vi "Experiment header-bundle parameters section wise.vi"(6 "Logging queue element":T1={"Imaging Protocol"=enum."Live Imaging", "Number of Trials"=0, "Frame Size"=100, "# Averaged frames"=0, "Dwell time (us)"=0.1, "Index of Z-plane"=0, "Timelapse?"=FALSE, "Logging process is active"=FALSE, "Speed logging enabled"=FALSE, "tdms file ref"=refnum, "path"=path "", "Trial Number"=0, "Expected # points acquired"=FALSE, "Manually stopped"=FALSE, "Last trial"=FALSE, "Ch0 data"=[], "Ch1 data"=[], "Ref Data"=[], "Ref Frame Time"=[], "Image Time"=[], "Continuous Time"=[], "Ref X Length"=0, "Ref Y Length"=0, "# Ref Averaged frames"=0, "Ref Dwell time (us)"=0.0, "Points acquired"={"Ch0 last trial"=0, "Ch1 last trial"=0, "All trials"=0}, "HW Timings File"=refnum} {"Ref Dwell time (us)" format="%#.6g"; "Frame Size" items=["100X100"=100, "128X128"=128, "200X200"=200, "256X256"=256, "512X512"=512, "1024x1024"=1024, "2048x2048"=2048]; "Dwell time (us)" format="%#.6g"}, 7 "Update header\ninterface cluster ?":bool, 8 "error in (no error)":errorcluster, 9 "Experiment data folder path":path, 10 "AOL_Globals":T25={"Imaging Protocol"=enum."AOL Z-Stack", "Number of POI"=0, "Number of Miniscans"=0, "Number of Trials"=0, "Number of Cycles "=0, "# Averaged Frames"=0, "Laser power (%)"=0, "Pockels (V)"=0.0, "Acquisition Length (sec)"=0.0, "Fill time (us)"=0.0, "POI Dwell time (us)"=0.0, "Miniscan Dwell time per pixel (us)"=0.0, "PMT 1"=0.0, "PMT 2"=0.0, "Back Apperture (mA)"=200.0, "Frame Size"=0, "Center Frequency"=0.0, "Field of View (um)"=175.0, "Field of View (norm)"=0.0, "DwellTime (us)"=0.0, "Ref Dwell Time (us)"=0.0, "Wavelength (nm)"=0.0, "Zoom"=0.0, "AOL Z"=0.0, "AOL Mode"=enum."Raster", "GridXY"=0.0, "GridZ"=0.0, "TriggerPeriod (sec)"=0.0, "Number of Pixels in Miniscan"=0, "Experiment folder path"=path "", "X centre"=0.0, "Y centre"=0.0, "Angle (degrees)"=0.0, "Angle Xs (degrees)"=0.0, "Angle Ys (degrees)"=0.0, "Plane Mode"=0, "Threshold"=[], "Regenerate Chirps"=FALSE, "Rectangle ROI length (pixels)"=0, "Rectangle ROI height (pixels)"=0, "AOD fill"=4900, "StartupDelay"=0, "Samples Wait after Trigger"=5080, "Slip Cycle"=600000, "Add Cycle"=TRUE, "Functional Mode"=enum."Point", "Z Start"=0.0, "Z Stop"=0.0, "# Planes"=0, "Total Pixels"=0, "Variable Miniscan Pixels"=[], "Use Variable Length"=FALSE, "Use Variable Resolution"=FALSE, "Laser power (%) at Z Start"=0, "Laser power (%) at Z Stop"=0, "Ref Z Step"=0} {"Angle Ys (degrees)" format="%#.6g"; "Angle Xs (degrees)" format="%#.6g"; "Plane Mode" items=["XY Plane", "XZ Plane", "YZ Plane", "arbitraryplane"]; "Frame Size" items=["100X100"=100, "128X128"=128, "200X200"=200, "256X256"=256, "512X512"=512, "1024x1024"=1024, "2048x2048"=2048]; "Back Apperture (mA)" format="%#.6g"; "Pockels (V)" format="%#.6g"; "PMT 2" format="%#.6g"; "PMT 1" format="%#.6g"; "Angle (degrees)" format="%#.6g"; "POI Dwell time (us)" format="%#.6g"}, 11 "Header file sections":T5=enum."GLOBAL PARAMETERS") -> (0 "error out":errorcluster, 3 "All header parameters in":T6 {"VOLUME IMAGING"."Plane Mode" items=["XY Plane", "XZ Plane", "YZ Plane", "arbitraryplane"]; "VOLUME IMAGING"."Basic Image meta data"."Frame Size" items=["100X100"=100, "128X128"=128, "200X200"=200, "256X256"=256, "512X512"=512, "1024x1024"=1024, "2048x2048"=2048]; "AOL Z-STACK"."Hdr Basic Image meta data"."Frame Size" items=["100X100"=100, "128X128"=128, "200X200"=200, "256X256"=256, "512X512"=512, "1024x1024"=1024, "2048x2048"=2048]; "MOTOR Z-STACK"."Hdr Basic Image meta data"."Frame Size" items=["100X100"=100, "128X128"=128, "200X200"=200, "256X256"=256, "512X512"=512, "1024x1024"=1024, "2048x2048"=2048]; "FUNCTIONAL IMAGING"."Plane Mode" items=["XY Plane", "XZ Plane", "YZ Plane", "arbitraryplane"]; "FUNCTIONAL IMAGING"."Basic Image meta data"."Frame Size" items=["100X100"=100, "128X128"=128, "200X200"=200, "256X256"=256, "512X512"=512, "1024x1024"=1024, "2048x2048"=2048]; "TIME SERIES"."Basic Image meta data"."Frame Size" items=["100X100"=100, "128X128"=128, "200X200"=200, "256X256"=256, "512X512"=512, "1024x1024"=1024, "2048x2048"=2048]})   [LabVIEW 2020]
uses:
  Typedefs/Controls/AOL_Globals.ctl
  Typedefs/Imaging Protocols enum.ctl
  Typedefs/Frame Size.ctl
  Typedefs/AOL modes.ctl
  Typedefs/Plane Mode.ctl
  Typedefs/Functional Mode.ctl
  Typedefs/Header parameters cluster-ALL.ctl
  Typedefs/Header subclusters/Header params -Login.ctl
  Typedefs/Header subclusters/Header params-Global Parameters.ctl
  Misc/Experiment Type.ctl
  Typedefs/Header subclusters/Header params-Imaging Modes.ctl
  Typedefs/Header subclusters/Header params-Time Series.ctl
  Typedefs/Header subclusters/Header params-Basic image meta data.ctl
  Typedefs/Header subclusters/Header params-Motor Z-stack.ctl
  Typedefs/Header subclusters/Header params-AOL Z-stack.ctl
  Typedefs/Header subclusters/Header params-Functional Imaging.ctl
  Typedefs/Header subclusters/Header params-Movement correction.ctl
  Typedefs/Reference source.ctl
  Typedefs/Header subclusters/Header params-Calibration Setup.ctl
  Typedefs/Header subclusters/Header params-statistics.ctl
  Misc/Biology Information.ctl
  Typedefs/Header subclusters/Header params-calibration data.ctl
  Typedefs/Header file sections.ctl
  Typedefs/Logging queue element.ctl
  Typedefs/Acquired points count.ctl
  ROI Entry screen/Typedefs/FGV ROI Time Ops.ctl
  Typedefs/Header file interface module functions enum.ctl
  Global Variables/General Globals.vi
  User profiles code/Globals/gl_UsrProfiles globals.vi
  Global Variables/gl_UI Ctrl Refs.vi
  Peripherals Control/Pockels/Globals/gl_Pockels control globals.vi
  Global Variables/gl_RefPlotRefreshRate.vi
  Configuration code/Calibration/Globals/gl_Calibration globals.vi
  Typedefs/Header subclusters/Header params-Volume Imaging.ctl
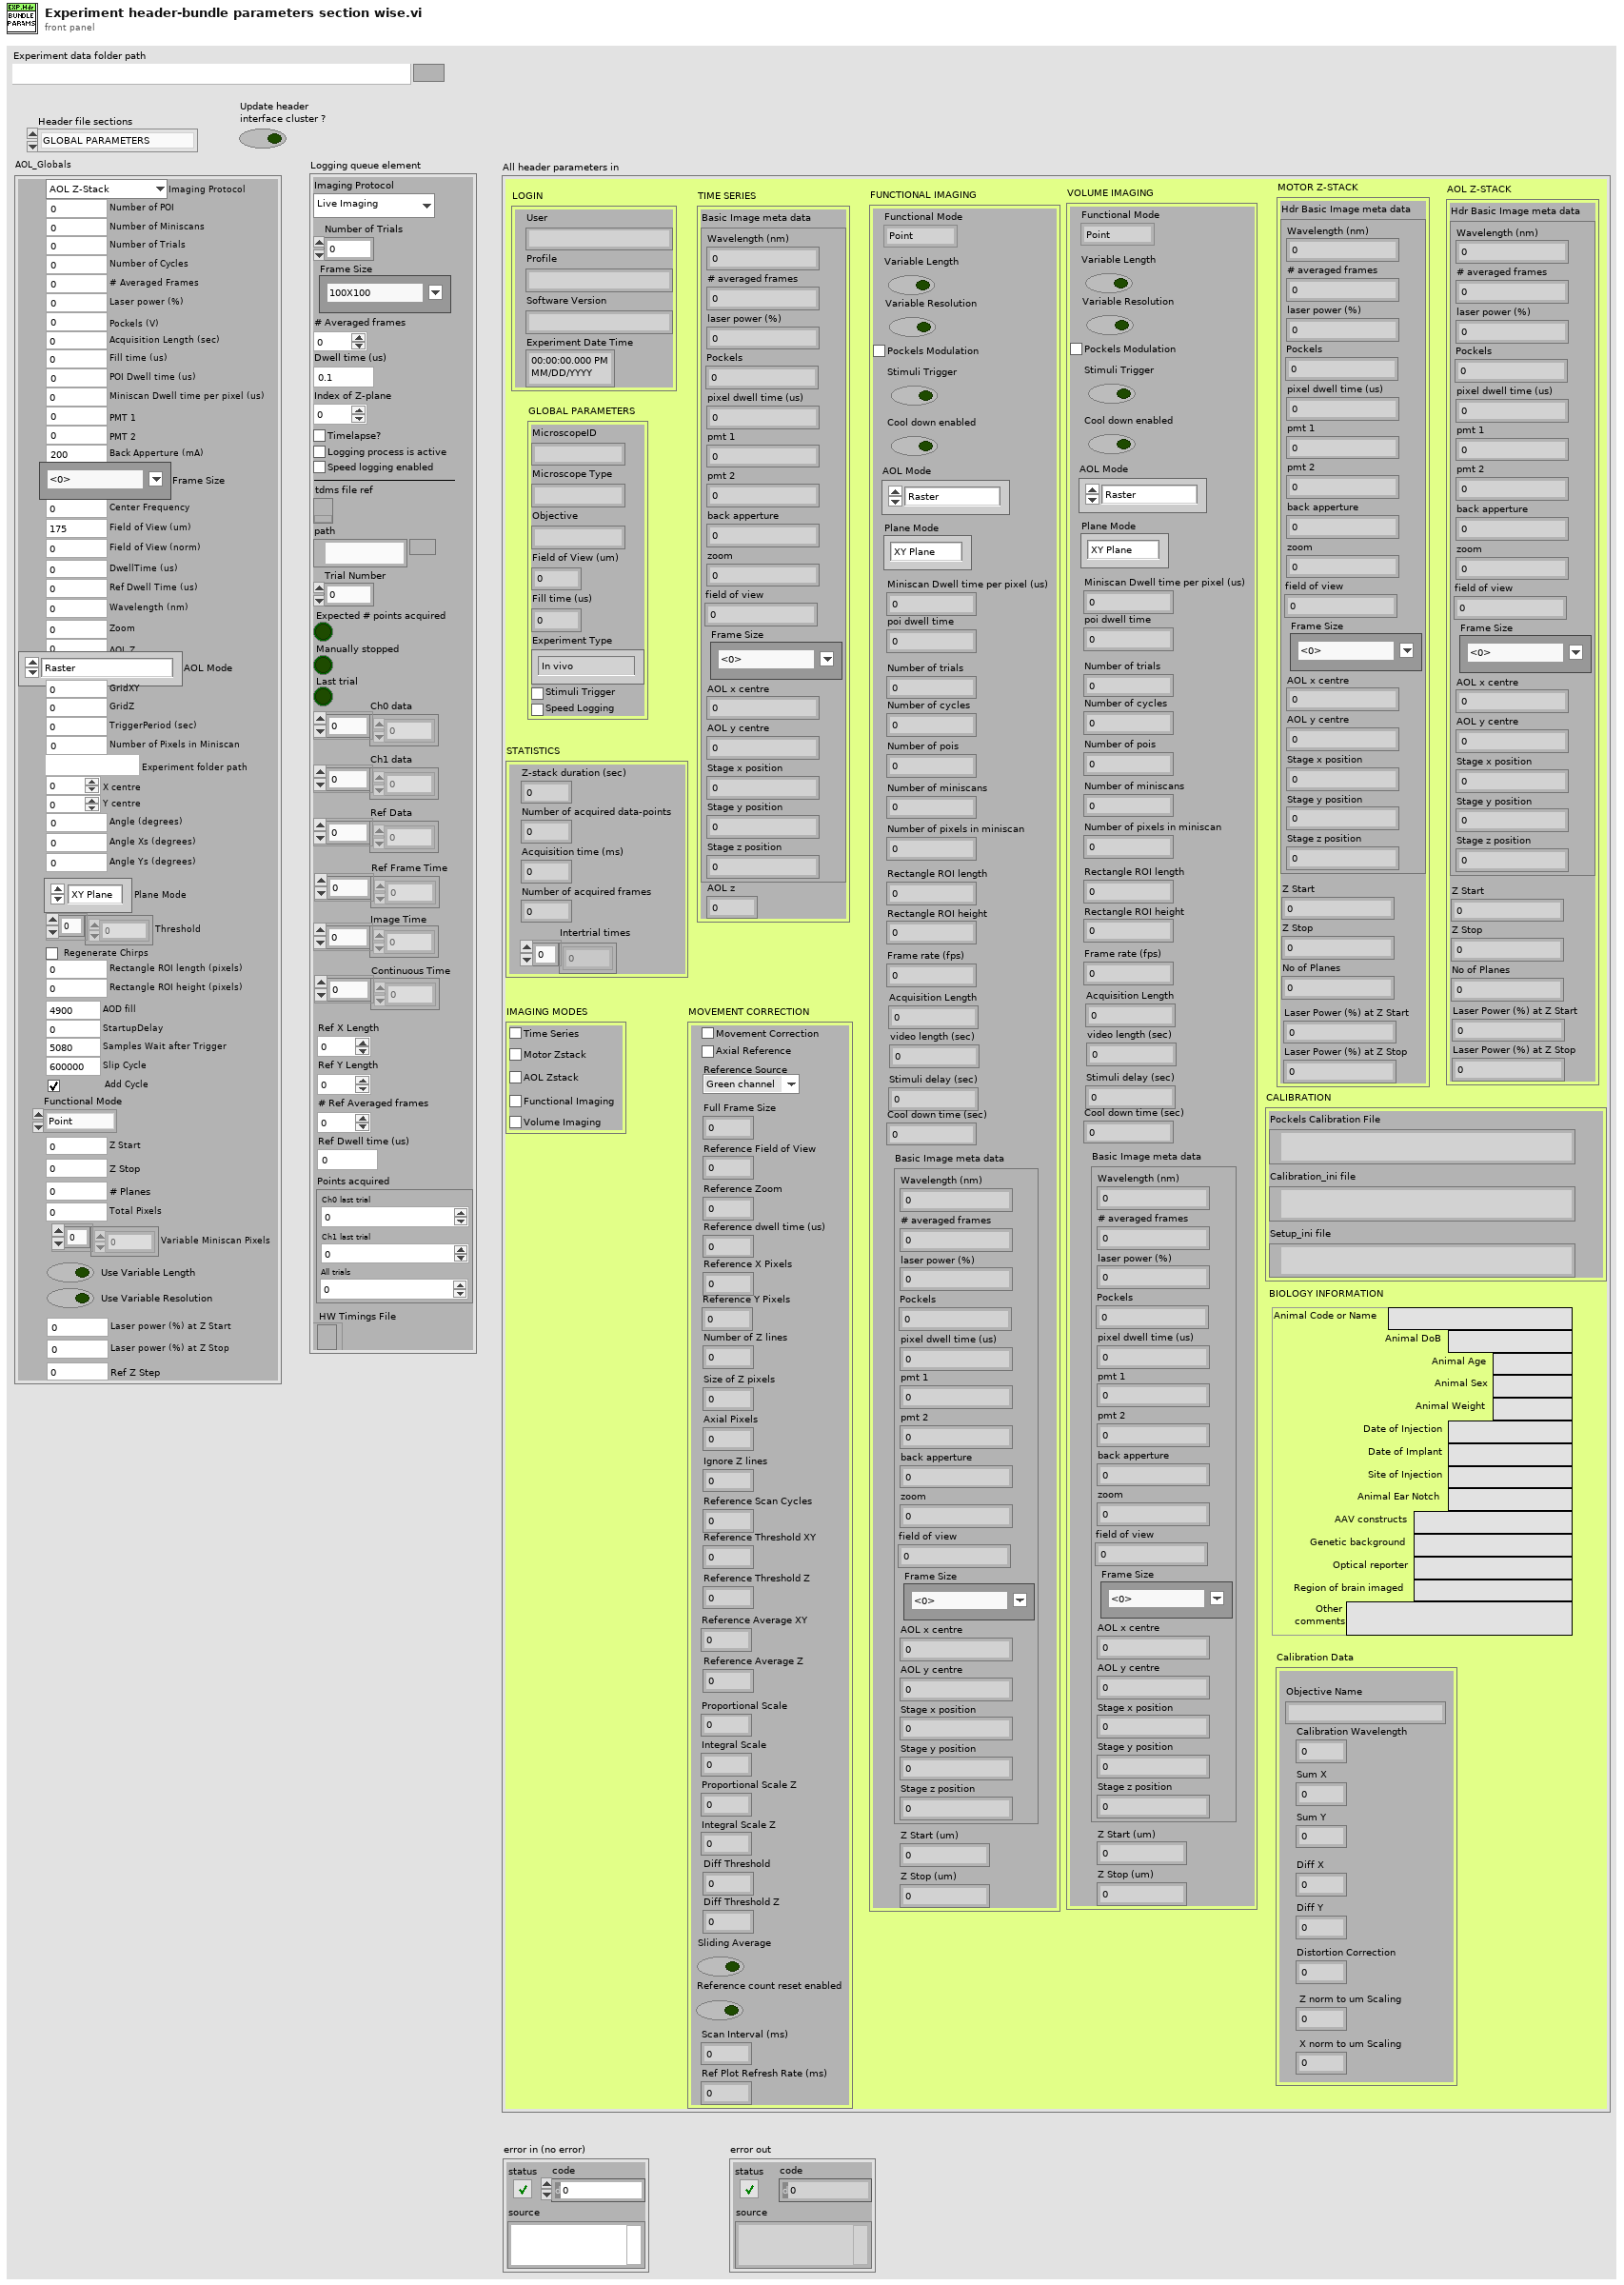
[diagram p1: front panel]
types:
  T1 = typedef "Logging queue element.ctl" = cluster{"Imaging Protocol":T2, "Number of Trials":u16, "Frame Size":T3, "# Averaged frames":u16, "Dwell time (us)":dbl, "Index of Z-plane":i32, "Timelapse?":bool, "Logging process is active":bool, "Speed logging enabled":bool, "tdms file ref":refnum<k34>, "path":path, "Trial Number":i32, "Expected # points acquired":bool, "Manually stopped":bool, "Last trial":bool, "Ch0 data":u32[], "Ch1 data":u32[], "Ref Data":u32[], "Ref Frame Time":u64[], "Image Time":u64[], "Continuous Time":u64[], "Ref X Length":u16, "Ref Y Length":u16, "# Ref Averaged frames":u16, "Ref Dwell time (us)":dbl, "Points acquired":T4, "HW Timings File":refnum<file>}
  T2 = typedef "Imaging Protocols enum.ctl" = enum16{"AOL Z-Stack", "Motor Z Stack", "Parameter Sweep", "Functional Acquisition", "Single Plane Acquisition", "Volume Acquisition", "Live Imaging", "Live Plane Imaging", "Live Volume Imaging"}
  T3 = typedef "Frame Size.ctl" = u16
  T4 = typedef "Acquired points count.ctl" = cluster{"Ch0 last trial":u64, "Ch1 last trial":u64, "All trials":u64}
  T5 = typedef "Header file sections.ctl" = enum16{"ALL SECTIONS", "LOGIN", "GLOBAL PARAMETERS", "CALIBRATION DATA", "IMAGING MODES", "TIME SERIES", "MOTOR Z-STACK", "AOL Z-STACK", "FUNCTIONAL IMAGING", "VOLUME IMAGING", "MOVEMENT CORRECTION", "CALIBRATION", "STATISTICS", "BIOLOGY INFORMATION"}
  T6 = typedef "Header parameters cluster-ALL.ctl" = cluster{"LOGIN":T7, "GLOBAL PARAMETERS":T8, "IMAGING MODES":T10, "TIME SERIES":T11, "MOTOR Z-STACK ":T13, "AOL Z-STACK":T14, "FUNCTIONAL IMAGING":T15, "VOLUME IMAGING":T15, "MOVEMENT CORRECTION":T19, "CALIBRATION":T21, "STATISTICS":T22, "BIOLOGY INFORMATION":T23, "Calibration Data":T24}
  T7 = typedef "Header params -Login.ctl" = cluster{"User":string, "Profile":string, "Software Version":string, "Experiment Date Time":timestamp}
  T8 = typedef "Header params-Global Parameters.ctl" = cluster{"MicroscopeID":string, "Microscope Type":string, "Objective":string, "Field of View (um)":dbl, "Fill time (us)":dbl, "Experiment Type":T9, "Stimuli Trigger":bool, "Speed Logging":bool}
  T9 = typedef "Experiment Type.ctl" = enum16{"In vivo", "In vitro", "Testing", "Calibration", "Other"}
  T10 = typedef "Header params-Imaging Modes.ctl" = cluster{"Time Series":bool, "Motor Zstack":bool, "AOL Zstack":bool, "Functional Imaging":bool, "Volume Imaging":bool}
  T11 = typedef "Header params-Time Series.ctl" = cluster{"Basic Image meta data":T12, "AOL z":dbl}
  T12 = typedef "Header params-Basic image meta data.ctl" = cluster{"Wavelength (nm)":dbl, "# averaged frames":dbl, "laser power (%)":dbl, "Pockels":dbl, "pixel dwell time (us)":dbl, "pmt 1":dbl, "pmt 2":dbl, "back apperture":dbl, "zoom":dbl, "field of view":dbl, "Frame Size":T3, "AOL x centre":dbl, "AOL y centre":dbl, "Stage x position":dbl, "Stage y position":dbl, "Stage z position":dbl}
  T13 = typedef "Header params-Motor Z-stack.ctl" = cluster{"Hdr Basic Image meta data":T12, "Z Start":dbl, "Z Stop":dbl, "No of Planes":i32, "Laser Power (%) at Z Start":dbl, "Laser Power (%) at Z Stop":dbl}
  T14 = typedef "Header params-AOL Z-stack.ctl" = cluster{"Hdr Basic Image meta data":T12, "Z Start":dbl, "Z Stop":dbl, "No of Planes":i32, "Laser Power (%) at Z Start":dbl, "Laser Power (%) at Z Stop":dbl}
  T15 = typedef "Header params-Functional Imaging.ctl" = cluster{"Functional Mode":T16, "Variable Length":bool, "Variable Resolution":bool, "Pockels Modulation":bool, "Stimuli Trigger":bool, "Cool down enabled":bool, "AOL Mode":T17, "Plane Mode":T18, "Miniscan Dwell time per pixel (us)":dbl, "poi dwell time":dbl, "Number of trials":dbl, "Number of cycles":dbl, "Number of pois":dbl, "Number of miniscans":dbl, "Number of pixels in miniscan":dbl, "Rectangle ROI length":dbl, "Rectangle ROI height":dbl, "Frame rate (fps)":dbl, "Acquisition Length":dbl, "video length (sec)":dbl, "Stimuli delay (sec)":dbl, "Cool down time (sec)":dbl, "Basic Image meta data":T12, "Z Start (um)":dbl, "Z Stop (um)":dbl}
  T16 = typedef "Functional Mode.ctl" = enum16{"Point", "Line", "Patch", "Plane", "Volume"}
  T17 = typedef "AOL modes.ctl" = enum16{"Raster", "Structural", "Pointing", "Mini Scan", "Alignment"}
  T18 = typedef "Plane Mode.ctl" = u16
  T19 = typedef "Header params-Movement correction.ctl" = cluster{"Movement Correction":bool, "Axial Reference":bool, "Reference Source":T20, "Full Frame Size":dbl, "Reference Field of View":dbl, "Reference Zoom":dbl, "Reference dwell time (us)":dbl, "Reference X Pixels":dbl, "Reference Y Pixels":dbl, "Number of Z lines":dbl, "Size of Z pixels":dbl, "Axial Pixels":dbl, "Ignore Z lines":dbl, "Reference Scan Cycles":dbl, "Reference Threshold XY":dbl, "Reference Threshold Z":dbl, "Reference Average XY":dbl, "Reference Average Z":dbl, "Proportional Scale":dbl, "Integral Scale":dbl, "Proportional Scale Z":dbl, "Integral Scale Z":dbl, "Diff Threshold":dbl, "Diff Threshold Z":dbl, "Sliding Average":bool, "Reference count reset enabled":bool, "Scan Interval (ms)":dbl, "Ref Plot Refresh Rate (ms)":dbl}
  T20 = typedef "Reference source.ctl" = enum16{"Green channel", "Red channel"}
  T21 = typedef "Header params-Calibration Setup.ctl" = cluster{"Pockels Calibration File":path, "Calibration_ini file":path, "Setup_ini file":path}
  T22 = typedef "Header params-statistics.ctl" = cluster{"Z-stack duration (sec)":dbl, "Number of acquired data-points":dbl, "Acquisition time (ms)":dbl, "Number of acquired frames":dbl, "Intertrial times":dbl[]}
  T23 = typedef "Biology Information.ctl" = cluster{"Animal Code or Name":string, "Animal DoB":string, "Animal Age":string, "Animal Sex":string, "Animal Weight":string, "Date of Injection":string, "Date of Implant":string, "Site of Injection":string, "Animal Ear Notch":string, "AAV constructs":string, "Genetic background":string, "Optical reporter":string, "Region of brain imaged":string, "Other \ncomments":string}
  T24 = typedef "Header params-calibration data.ctl" = cluster{"Objective Name":string, "Calibration Wavelength":dbl, "Sum X":dbl, "Sum Y":dbl, "Diff X":dbl, "Diff Y":dbl, "Distortion Correction":dbl, " Z norm to um Scaling":dbl, " X norm to um Scaling":dbl}
  T25 = typedef "AOL_Globals.ctl" = cluster{"Imaging Protocol":T2, "Number of POI":u16, "Number of Miniscans":u16, "Number of Trials":u16, "Number of Cycles ":u64, "# Averaged Frames":u16, "Laser power (%)":u8, "Pockels (V)":dbl, "Acquisition Length (sec)":dbl, "Fill time (us)":dbl, "POI Dwell time (us)":dbl, "Miniscan Dwell time per pixel (us)":dbl, "PMT 1":dbl, "PMT 2":dbl, "Back Apperture (mA)":dbl, "Frame Size":T3, "Center Frequency":dbl, "Field of View (um)":dbl, "Field of View (norm)":dbl, "DwellTime (us)":dbl, "Ref Dwell Time (us)":dbl, "Wavelength (nm)":dbl, "Zoom":dbl, "AOL Z":dbl, "AOL Mode":T17, "GridXY":dbl, "GridZ":dbl, "TriggerPeriod (sec)":dbl, "Number of Pixels in Miniscan":u16, "Experiment folder path":path, "X centre":dbl, "Y centre":dbl, "Angle (degrees)":dbl, "Angle Xs (degrees)":dbl, "Angle Ys (degrees)":dbl, "Plane Mode":T18, "Threshold":u16[], "Regenerate Chirps":bool, "Rectangle ROI length (pixels)":u16, "Rectangle ROI height (pixels)":u16, "AOD fill":u16, "StartupDelay":i32, "Samples Wait after Trigger":u16, "Slip Cycle":u32, "Add Cycle":bool, "Functional Mode":T16, "Z Start":dbl, "Z Stop":dbl, "# Planes":i32, "Total Pixels":i32, "Variable Miniscan Pixels":u16[], "Use Variable Length":bool, "Use Variable Resolution":bool, "Laser power (%) at Z Start":u8, "Laser power (%) at Z Stop":u8, "Ref Z Step":i8}
  T26 = typedef "FGV ROI Time Ops.ctl" = enum16{"Read", "Write Cycle Time", "Write Cycle Rate"}
  T27 = typedef "UI ctrl refs cluster.ctl" = cluster{"Top level VI path":path, "Top level VI ref":refnum<vi>, "User menu ref":refnum<k9>, "Sub Panel control":refnum<vi>, "Imaging Param Tab":refnum<vi>, "Occurrence-Start drivers":refnum<k4>, "Occurrence-Speed logging initialised":refnum<k4>, "Occurrence-XYZ stage initialised":refnum<k4>, "Exit button":refnum<vi>, "Status ind":refnum<vi>, "Set as origin":refnum<vi>, "Speed Logging":refnum<vi>, "Time Lapse":refnum<vi>, "Live Imaging":refnum<vi>, "AOL Z Stack":refnum<vi>, "Motor Z Stack":refnum<vi>, "Funct Acq button":refnum<vi>, "Hard Shutter":refnum<vi>, "Virtual Shutter":refnum<vi>, "Laser Power":refnum<vi>, "AOL Mode":refnum<vi>, "Frame Size":refnum<vi>, "Field of View":refnum<vi>, "Dwell Time":refnum<vi>, "Zoom":refnum<vi>, "AOL Z":refnum<vi>, "Objective":refnum<vi>, "Axis":refnum<vi>, "Paths & Names":refnum<vi>, "Experiment folder path (ind.)":refnum<vi>, "Last State (Ind.)":refnum<vi>, "Averages":refnum<vi>, "Angle (degrees)":refnum<vi>, "X centre":refnum<vi>, "Y centre":refnum<vi>, "Plane Mode":refnum<vi>, "# Planes":refnum<vi>, "Z Start":refnum<vi>, "Z Stop":refnum<vi>, "Z Step":refnum<vi>, "PMT 1":refnum<vi>, "PMT 2":refnum<vi>, "Stage XYZ Position":refnum<vi>, "Pockels@Z Start":refnum<vi>, "Pockels@Z Stop":refnum<vi>, "Obtain Z Start":refnum<vi>, "Obtain Z Stop":refnum<vi>, "Live stim.trig.period":refnum<vi>, "Live stim.trig.enable":refnum<vi>, "Movement Correction":refnum<vi>, "Load Reference Image":refnum<vi>, "XY Stage Move":refnum<vi>, "MovCor Cluster":refnum<vi>, "RefDAQParam":refnum<vi>, "Funct. Acq. Pockels Modulation":refnum<vi>, "Ref Laser Power":refnum<vi>, "Enable Video Recording":refnum<vi>, "Video Record-Live Imaging":refnum<vi>, "Video Record-Funct acq":refnum<vi>, "Reference Source":refnum<vi>, "AOL Z-stack Chirps Ready (ind)":refnum<vi>, "Target time between mov.cor. ref triggers (ms)":refnum<vi>, "Funct. Acq. Ref frame save":refnum<vi>, "Tracking button":refnum<vi>, "Show ref plots window":refnum<vi>, "Center freq ind (nm)":refnum<vi>, "Pickup mode (ind)":refnum<vi>, "Logging queue (ind)":refnum<vi>, "Back aperture power (ind.)":refnum<vi>, "Power after objective (ind.)":refnum<vi>, "Switch user":refnum<vi>, "Ls1 Conn. Status":refnum<vi>, "Ls1Tuning Status":refnum<vi>, "Ls1 Faults":refnum<vi>, "Ls1 Connection":refnum<vi>, "Ls1 Mode":refnum<vi>, "Ls1 POWER [mW]":refnum<vi>, "Ls1Shutter":refnum<vi>, "Ls1 Wavelength":refnum<vi>, "Ls1 Note":refnum<vi>, "Ls1 Confirm Wav":refnum<vi>, "Ls1 PreChrp Prism1":refnum<vi>, "Ls1 PreChrp Prism2":refnum<vi>, "Ls1 wav top Ind":refnum<vi>, "Ls1 power top Ind":refnum<vi>, "Ls1 Pump peak Hold":refnum<vi>, "Ls1 Status Ind":refnum<vi>, "Ls1 wav cancel":refnum<vi>, "Experiment Type":refnum<vi>, "Biology Information":refnum<vi>, "Camera recording status":refnum<vi>, "Optimise Obj. Pos.":refnum<vi>}
  T28 = typedef "Objective Config.ctl" = cluster{"Name":string, "Sum X":dbl, "Sum Y":dbl, "Diff X":dbl, "Diff Y":dbl, "Distortion Correction":dbl, "Z_norm to um_scaling":dbl, "X_norm to um_scaling":dbl, "Calibrated Wavelength":dbl}
  T29 = typedef "Header params-Volume Imaging.ctl" = cluster{"Functional Mode":T16, "Pockels Modulation":bool, "Number of pois":dbl, "Number of miniscans":dbl, "Number of cycles":dbl, "Number of trials":dbl, "Miniscan dwell time per pixel (us)":dbl, "Number of pixels in miniscan":dbl, "poi dwell time":dbl, "Rectangle ROI length":dbl, "Rectangle ROI height":dbl, "AOL Mode":T17, "Plane Mode":T18, "video length (sec)":dbl, "Frame rate (fps)":dbl, "Stimuli Timing (usec)":dbl, "Acquisition Length":dbl, "Basic Image meta data":T12, "Z Start (um)":dbl, "Z Stop (um)":dbl}
  T30 = typedef "Ref DAQ Param.ctl" = cluster{"Full Frame Size":u16, "Ref Field of View":sgl, "Ref Zoom":i8, "Ref_dwellTime":sgl, "Ref X-pixels-per-line(Npxr)":i16, "Ref Y-lines-per-image(Npyr)":i16, "Ref Z-lines-per-image":i16, "Ignore Z lines":i16, "Ref Scan Cycles":i32, "Ref threshold XY":u16, "Ref threshold Z":u16, "Ref average XY":u16, "Ref Average  Z":u16, "Proportional_scale":fxp<+,16,2>, "Integral_scale":fxp<+/-,16,12>, "Proportional_scale Z":fxp<+,16,2>, "Integral_scale Z":fxp<+/-,16,12>, "Diff_threshold":fxp<+,16,2>, "Diff_threshold _z":fxp<+,16,2>, "Sliding Average":bool, "Ref count reset enabled":bool, "Auto-centering":bool}
  T31 = typedef "Reference_Globals.ctl" = cluster{"Refrence data path":path, "Reference Rectangle":i16[][], "AOL Z":dbl, "No of pixels in a miniscan ":i32[], "Threshold":i16[], "No of miniscans":i32[], "Full Frame Size":u16, "Reference Image":T32, "dwelltime":dbl, "Zoom":dbl, "Field of View":dbl, "Z Step":i8, "Z pixels":i32, "Z Lines":u8, "Z Ignore":u8, "Laser":u8, "Auto centering":bool}
  T32 = typedef "IMAQ Image.ctl" = refnum<image>
  T33 = typedef "Header file interface module functions enum.ctl" = enum16{"Load experiment header file", "Save experiment header file", "Clear stored values", "Read stored values", "Update specific value in memory", "Update values in memory"}
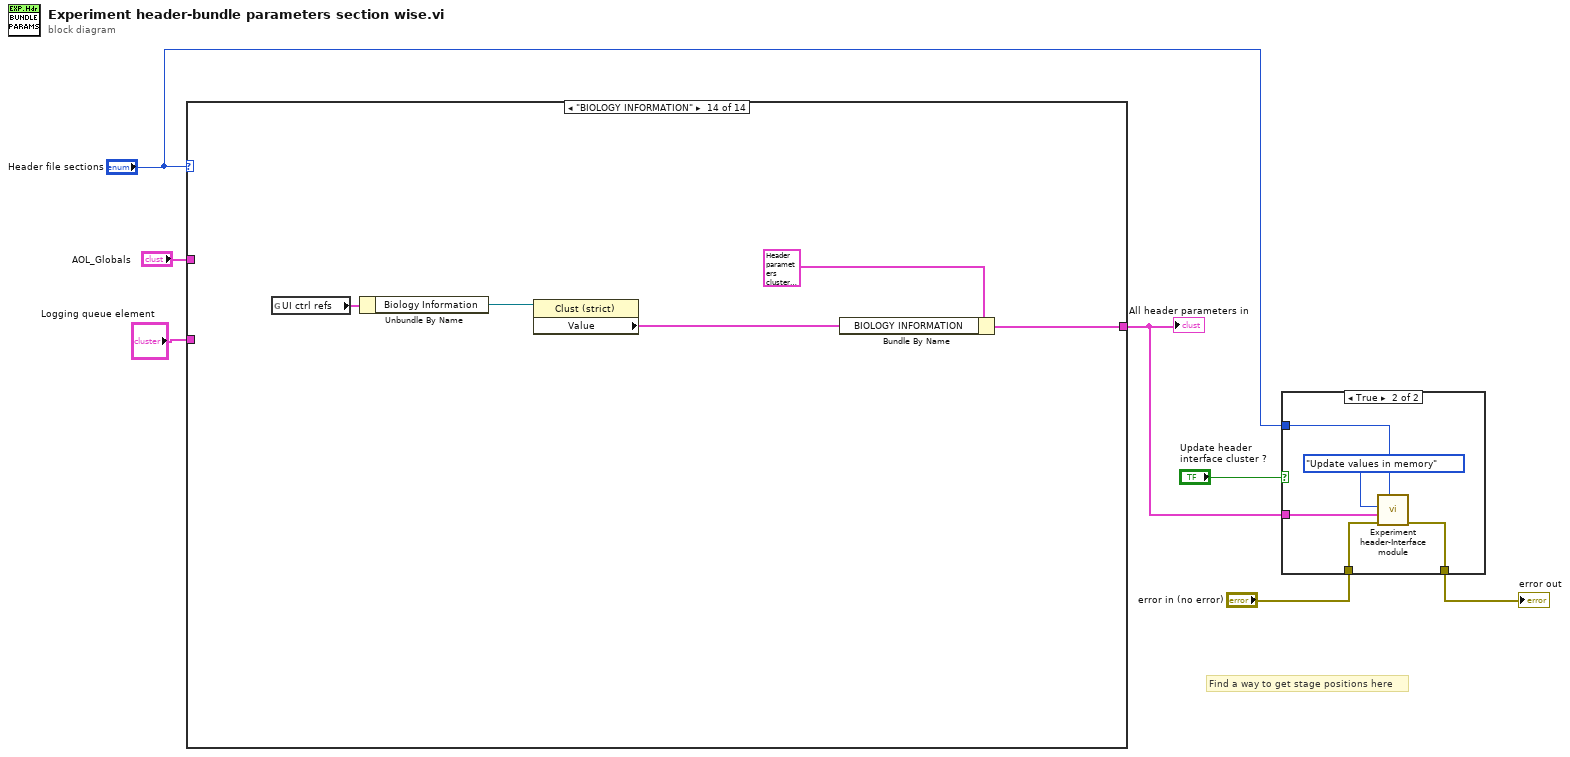
[diagram p0: block diagram]
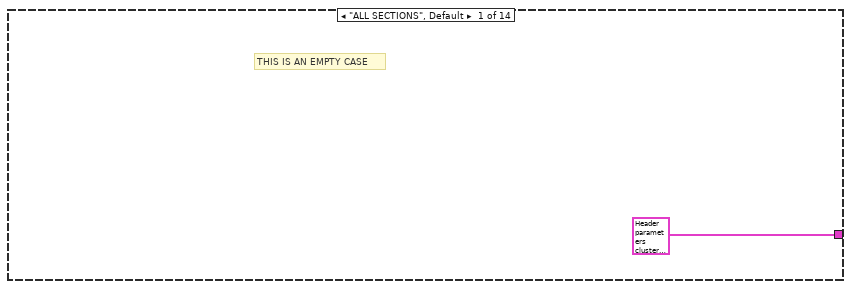
[diagram p3: hidden frame]
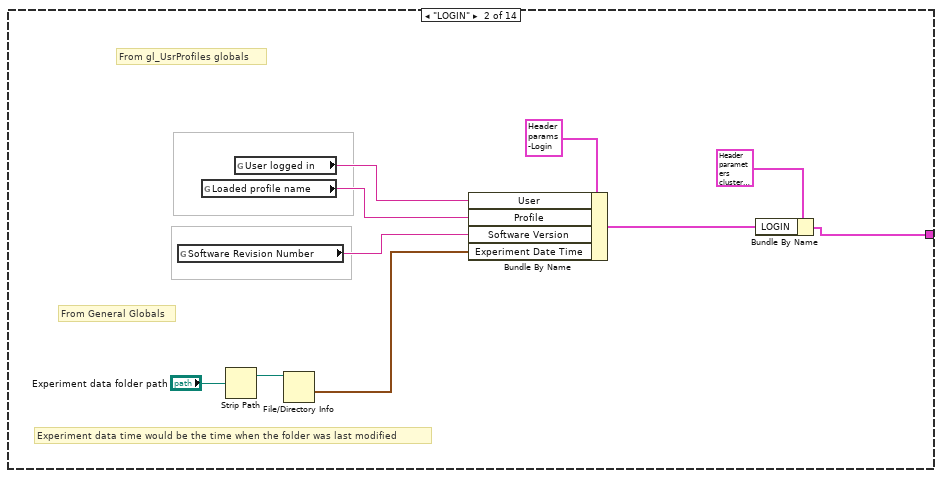
[diagram p4: hidden frame]
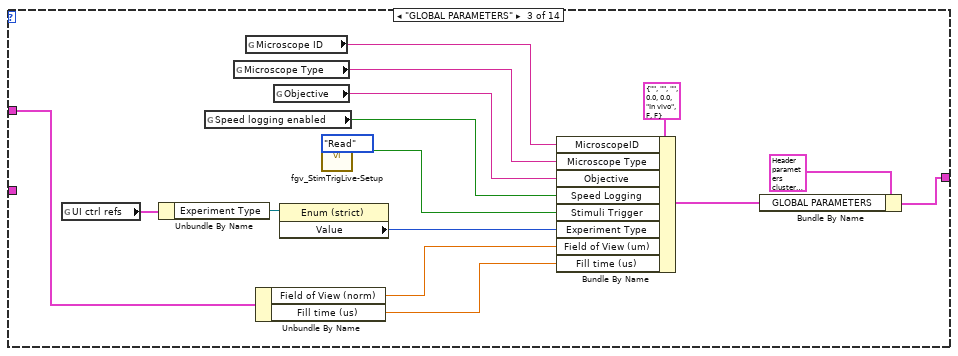
[diagram p5: hidden frame]
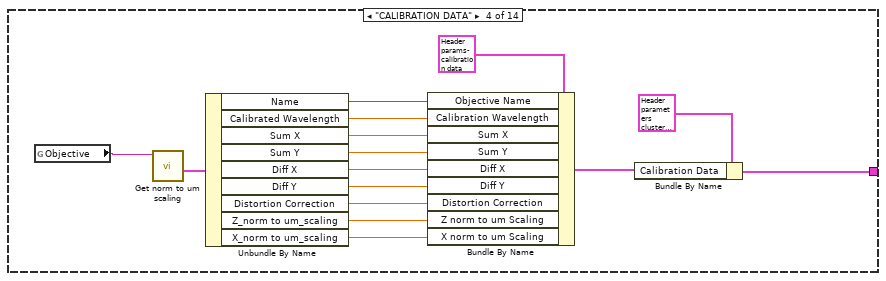
[diagram p6: hidden frame]
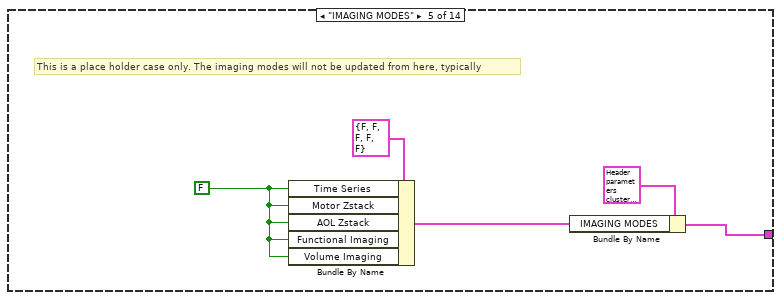
[diagram p7: hidden frame]
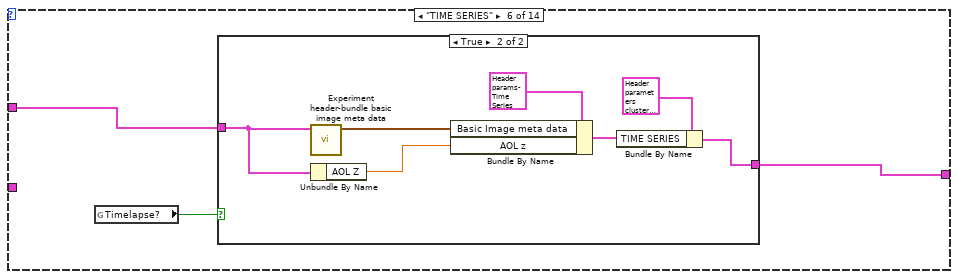
[diagram p8: hidden frame]
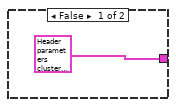
[diagram p9: hidden frame]
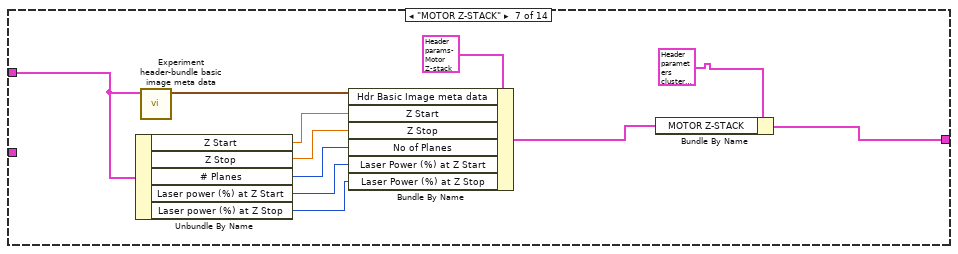
[diagram p10: hidden frame]
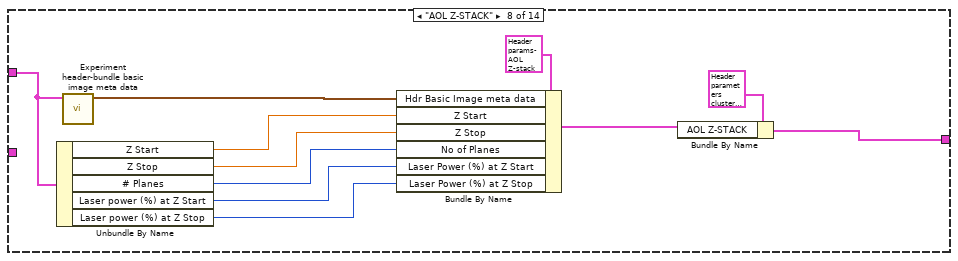
[diagram p11: hidden frame]
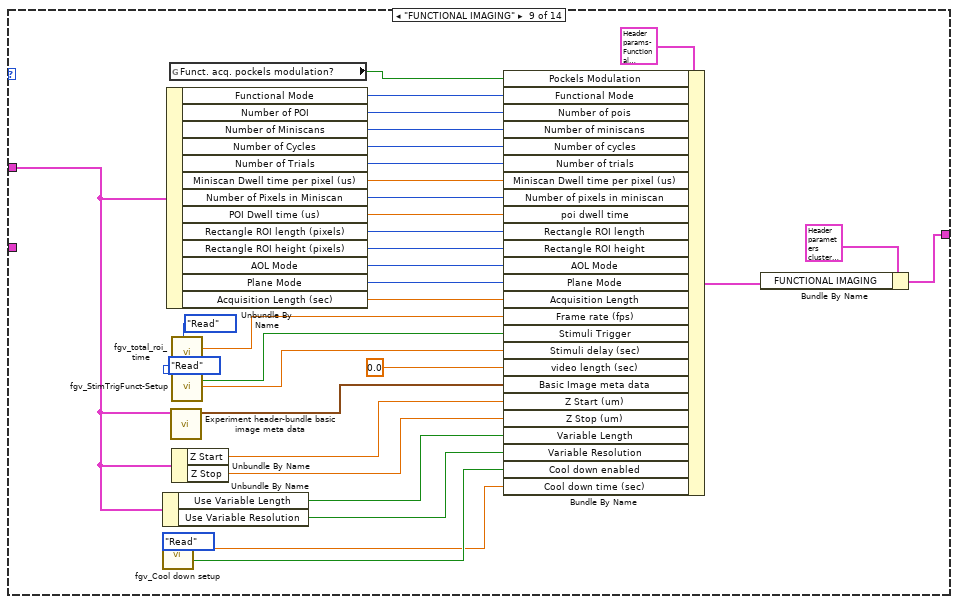
[diagram p12: hidden frame]
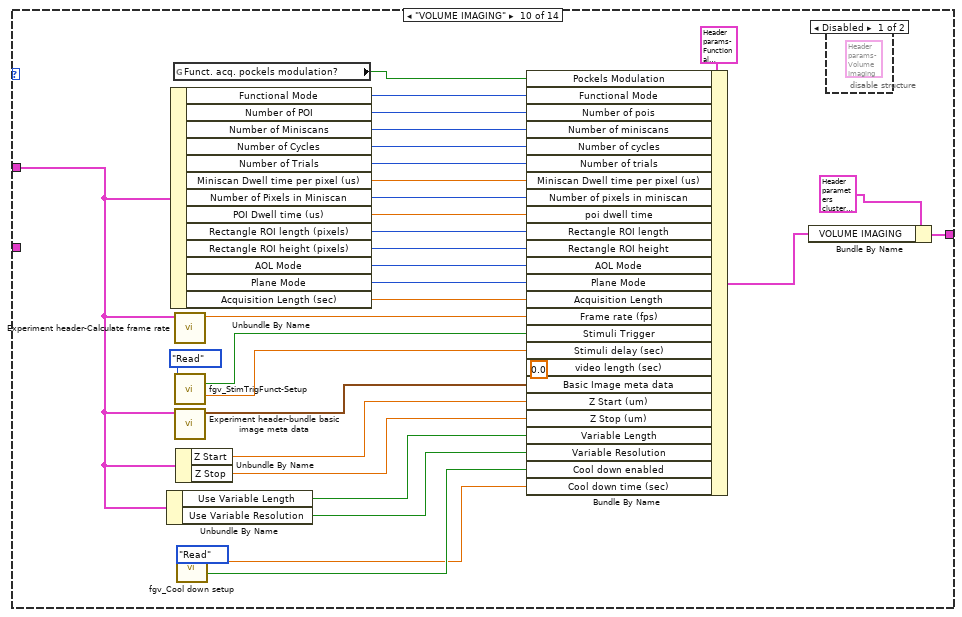
[diagram p13: hidden frame]
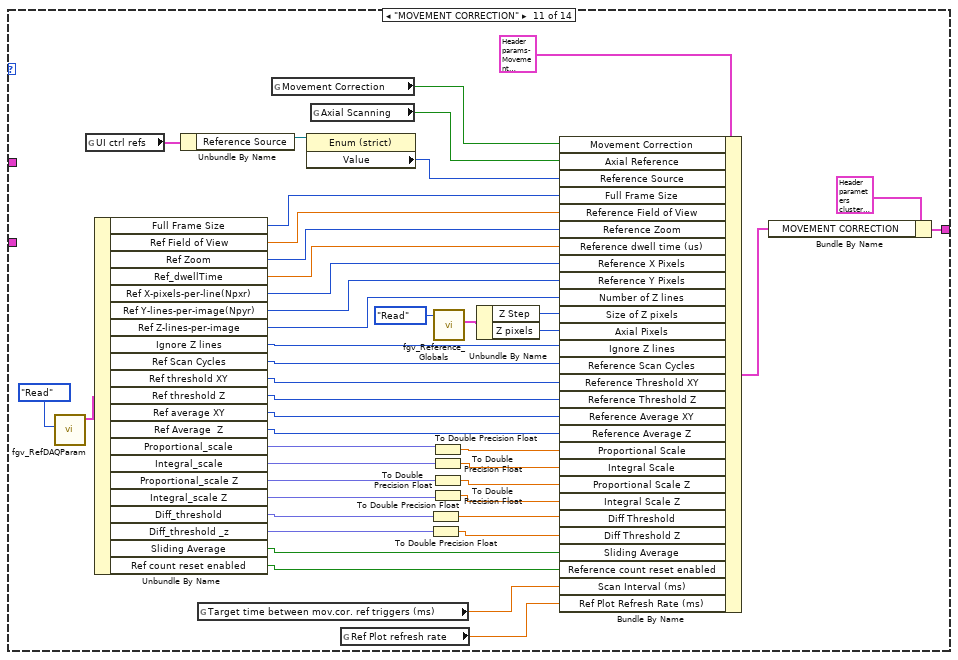
[diagram p15: hidden frame]
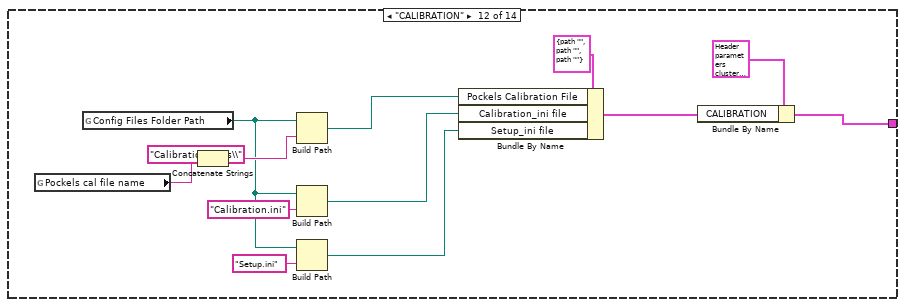
[diagram p16: hidden frame]
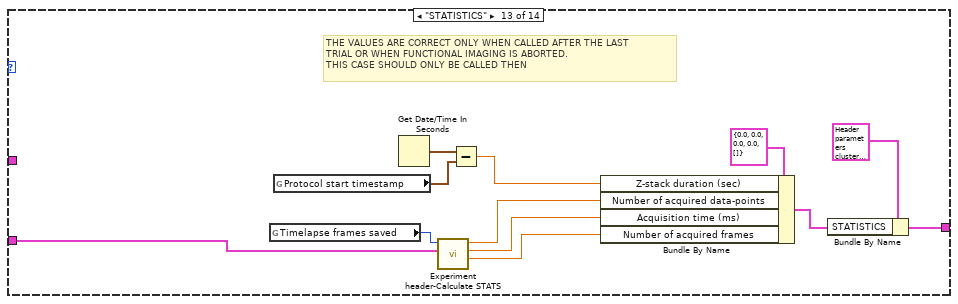
[diagram p17: hidden frame]
diagram:
  # "Find a way to get stage positions here"
  n1 = case shown="\"BIOLOGY INFORMATION\"" "Header file sections" {
    tunnel: "AOL_Globals" -> [_ _ w30 _ _ w56 w72 w83 w99 w130 _ _ _ _]
    tunnel: [T6 {"LOGIN"={"User"="", "Profile"="", "Software Version"="", "Experiment Date Time"=timestamp(0 s since 1904-01-01)}, "GLOBAL PARAMETERS"={"MicroscopeID"="", "Microscope Type"="", "Objective"="", "Field of View (um)"=0.0, "Fill time (us)"=0.0, "Experiment Type"=enum."In vivo", "Stimuli Trigger"=FALSE, "Speed Logging"=FALSE}, "IMAGING MODES"={"Time Series"=FALSE, "Motor Zstack"=FALSE, "AOL Zstack"=FALSE, "Functional Imaging"=FALSE, "Volume Imaging"=FALSE}, "TIME SERIES"={"Basic Image meta data"={"Wavelength (nm)"=0.0, "# averaged frames"=0.0, "laser power (%)"=0.0, "Pockels"=0.0, "pixel dwell time (us)"=0.0, "pmt 1"=0.0, "pmt 2"=0.0, "back apperture"=0.0, "zoom"=0.0, "field of view"=0.0, "Frame Size"=0, "AOL x centre"=0.0, "AOL y centre"=0.0, "Stage x position"=0.0, "Stage y position"=0.0, "Stage z position"=0.0}, "AOL z"=0.0}, "MOTOR Z-STACK "={"Hdr Basic Image meta data"={"Wavelength (nm)"=0.0, "# averaged frames"=0.0, "laser power (%)"=0.0, "Pockels"=0.0, "pixel dwell time (us)"=0.0, "pmt 1"=0.0, "pmt 2"=0.0, "back apperture"=0.0, "zoom"=0.0, "field of view"=0.0, "Frame Size"=0, "AOL x centre"=0.0, "AOL y centre"=0.0, "Stage x position"=0.0, "Stage y position"=0.0, "Stage z position"=0.0}, "Z Start"=0.0, "Z Stop"=0.0, "No of Planes"=0, "Laser Power (%) at Z Start"=0.0, "Laser Power (%) at Z Stop"=0.0}, "AOL Z-STACK"={"Hdr Basic Image meta data"={"Wavelength (nm)"=0.0, "# averaged frames"=0.0, "laser power (%)"=0.0, "Pockels"=0.0, "pixel dwell time (us)"=0.0, "pmt 1"=0.0, "pmt 2"=0.0, "back apperture"=0.0, "zoom"=0.0, "field of view"=0.0, "Frame Size"=0, "AOL x centre"=0.0, "AOL y centre"=0.0, "Stage x position"=0.0, "Stage y position"=0.0, "Stage z position"=0.0}, "Z Start"=0.0, "Z Stop"=0.0, "No of Planes"=0, "Laser Power (%) at Z Start"=0.0, "Laser Power (%) at Z Stop"=0.0}, "FUNCTIONAL IMAGING"={"Functional Mode"=enum."Point", "Variable Length"=FALSE, "Variable Resolution"=FALSE, "Pockels Modulation"=FALSE, "Stimuli Trigger"=FALSE, "Cool down enabled"=FALSE, "AOL Mode"=enum."Raster", "Plane Mode"=0, "Miniscan Dwell time per pixel (us)"=0.0, "poi dwell time"=0.0, "Number of trials"=0.0, "Number of cycles"=0.0, "Number of pois"=0.0, "Number of miniscans"=0.0, "Number of pixels in miniscan"=0.0, "Rectangle ROI length"=0.0, "Rectangle ROI height"=0.0, "Frame rate (fps)"=0.0, "Acquisition Length"=0.0, "video length (sec)"=0.0, "Stimuli delay (sec)"=0.0, "Cool down time (sec)"=0.0, "Basic Image meta data"={"Wavelength (nm)"=0.0, "# averaged frames"=0.0, "laser power (%)"=0.0, "Pockels"=0.0, "pixel dwell time (us)"=0.0, "pmt 1"=0.0, "pmt 2"=0.0, "back apperture"=0.0, "zoom"=0.0, "field of view"=0.0, "Frame Size"=0, "AOL x centre"=0.0, "AOL y centre"=0.0, "Stage x position"=0.0, "Stage y position"=0.0, "Stage z position"=0.0}, "Z Start (um)"=0.0, "Z Stop (um)"=0.0}, "VOLUME IMAGING"={"Functional Mode"=enum."Point", "Variable Length"=FALSE, "Variable Resolution"=FALSE, "Pockels Modulation"=FALSE, "Stimuli Trigger"=FALSE, "Cool down enabled"=FALSE, "AOL Mode"=enum."Raster", "Plane Mode"=0, "Miniscan Dwell time per pixel (us)"=0.0, "poi dwell time"=0.0, "Number of trials"=0.0, "Number of cycles"=0.0, "Number of pois"=0.0, "Number of miniscans"=0.0, "Number of pixels in miniscan"=0.0, "Rectangle ROI length"=0.0, "Rectangle ROI height"=0.0, "Frame rate (fps)"=0.0, "Acquisition Length"=0.0, "video length (sec)"=0.0, "Stimuli delay (sec)"=0.0, "Cool down time (sec)"=0.0, "Basic Image meta data"={"Wavelength (nm)"=0.0, "# averaged frames"=0.0, "laser power (%)"=0.0, "Pockels"=0.0, "pixel dwell time (us)"=0.0, "pmt 1"=0.0, "pmt 2"=0.0, "back apperture"=0.0, "zoom"=0.0, "field of view"=0.0, "Frame Size"=0, "AOL x centre"=0.0, "AOL y centre"=0.0, "Stage x position"=0.0, "Stage y position"=0.0, "Stage z position"=0.0}, "Z Start (um)"=0.0, "Z Stop (um)"=0.0}, "MOVEMENT CORRECTION"={"Movement Correction"=FALSE, "Axial Reference"=FALSE, "Reference Source"=enum."Green channel", "Full Frame Size"=0.0, "Reference Field of View"=0.0, "Reference Zoom"=0.0, "Reference dwell time (us)"=0.0, "Reference X Pixels"=0.0, "Reference Y Pixels"=0.0, "Number of Z lines"=0.0, "Size of Z pixels"=0.0, "Axial Pixels"=0.0, "Ignore Z lines"=0.0, "Reference Scan Cycles"=0.0, "Reference Threshold XY"=0.0, "Reference Threshold Z"=0.0, "Reference Average XY"=0.0, "Reference Average Z"=0.0, "Proportional Scale"=0.0, "Integral Scale"=0.0, "Proportional Scale Z"=0.0, "Integral Scale Z"=0.0, "Diff Threshold"=0.0, "Diff Threshold Z"=0.0, "Sliding Average"=FALSE, "Reference count reset enabled"=FALSE, "Scan Interval (ms)"=0.0, "Ref Plot Refresh Rate (ms)"=0.0}, "CALIBRATION"={"Pockels Calibration File"=path "", "Calibration_ini file"=path "", "Setup_ini file"=path ""}, "STATISTICS"={"Z-stack duration (sec)"=0.0, "Number of acquired data-points"=0.0, "Acquisition time (ms)"=0.0, "Number of acquired frames"=0.0, "Intertrial times"=[]}, "BIOLOGY INFORMATION"={"Animal Code or Name"="", "Animal DoB"="", "Animal Age"="", "Animal Sex"="", "Animal Weight"="", "Date of Injection"="", "Date of Implant"="", "Site of Injection"="", "Animal Ear Notch"="", "AAV constructs"="", "Genetic background"="", "Optical reporter"="", "Region of brain imaged"="", "Other \ncomments"=""}, "Calibration Data"={"Objective Name"="", "Calibration Wavelength"=0.0, "Sum X"=0.0, "Sum Y"=0.0, "Diff X"=0.0, "Diff Y"=0.0, "Distortion Correction"=0.0, " Z norm to um Scaling"=0.0, " X norm to um Scaling"=0.0}} ("All header parameters in") w13 w20 w36 w52 w57 w73 w85 w118 w151 w192 w198 w221 w223] -> w1
    tunnel: "Logging queue element" -> [_ _ _ _ _ _ _ _ _ _ _ _ w219 _]
    frame "ALL SECTIONS", Default {
      # "THIS IS AN EMPTY CASE"
    }
    frame "LOGIN" {
      # "Experiment data time would be the time when the folder was last modified"
      # "From General Globals"
      # "From gl_UsrProfiles globals"
      n2 = global read "General Globals.vi" "Software Revision Number"() -> (w15:string)
      n3 = global read "gl_UsrProfiles globals.vi" "Loaded profile name"() -> (w16:string)
      n4 = Strip Path(path="Experiment data folder path") -> (stripped path=w11:path)  [unwired: 1 out]
      n5 = global read "gl_UsrProfiles globals.vi" "User logged in"() -> (w17:string)
      n6 = File/Directory Info(path=w11) -> (last mod=w10:timestamp)  [unwired: 1 in, 6 out]
      n7 = Bundle By Name(cluster=T7 {"User"="", "Profile"="", "Software Version"="", "Experiment Date Time"=timestamp(0 s since 1904-01-01)} ("LOGIN"), "User"=w17, "Profile"=w16, "Software Version"=w15, "Experiment Date Time"=w10) -> (w14:T7)
      n8 = Bundle By Name(cluster=T6 {"LOGIN"={"User"="", "Profile"="", "Software Version"="", "Experiment Date Time"=timestamp(0 s since 1904-01-01)}, "GLOBAL PARAMETERS"={"MicroscopeID"="", "Microscope Type"="", "Objective"="", "Field of View (um)"=0.0, "Fill time (us)"=0.0, "Experiment Type"=enum."In vivo", "Stimuli Trigger"=FALSE, "Speed Logging"=FALSE}, "IMAGING MODES"={"Time Series"=FALSE, "Motor Zstack"=FALSE, "AOL Zstack"=FALSE, "Functional Imaging"=FALSE, "Volume Imaging"=FALSE}, "TIME SERIES"={"Basic Image meta data"={"Wavelength (nm)"=0.0, "# averaged frames"=0.0, "laser power (%)"=0.0, "Pockels"=0.0, "pixel dwell time (us)"=0.0, "pmt 1"=0.0, "pmt 2"=0.0, "back apperture"=0.0, "zoom"=0.0, "field of view"=0.0, "Frame Size"=0, "AOL x centre"=0.0, "AOL y centre"=0.0, "Stage x position"=0.0, "Stage y position"=0.0, "Stage z position"=0.0}, "AOL z"=0.0}, "MOTOR Z-STACK "={"Hdr Basic Image meta data"={"Wavelength (nm)"=0.0, "# averaged frames"=0.0, "laser power (%)"=0.0, "Pockels"=0.0, "pixel dwell time (us)"=0.0, "pmt 1"=0.0, "pmt 2"=0.0, "back apperture"=0.0, "zoom"=0.0, "field of view"=0.0, "Frame Size"=0, "AOL x centre"=0.0, "AOL y centre"=0.0, "Stage x position"=0.0, "Stage y position"=0.0, "Stage z position"=0.0}, "Z Start"=0.0, "Z Stop"=0.0, "No of Planes"=0, "Laser Power (%) at Z Start"=0.0, "Laser Power (%) at Z Stop"=0.0}, "AOL Z-STACK"={"Hdr Basic Image meta data"={"Wavelength (nm)"=0.0, "# averaged frames"=0.0, "laser power (%)"=0.0, "Pockels"=0.0, "pixel dwell time (us)"=0.0, "pmt 1"=0.0, "pmt 2"=0.0, "back apperture"=0.0, "zoom"=0.0, "field of view"=0.0, "Frame Size"=0, "AOL x centre"=0.0, "AOL y centre"=0.0, "Stage x position"=0.0, "Stage y position"=0.0, "Stage z position"=0.0}, "Z Start"=0.0, "Z Stop"=0.0, "No of Planes"=0, "Laser Power (%) at Z Start"=0.0, "Laser Power (%) at Z Stop"=0.0}, "FUNCTIONAL IMAGING"={"Functional Mode"=enum."Point", "Variable Length"=FALSE, "Variable Resolution"=FALSE, "Pockels Modulation"=FALSE, "Stimuli Trigger"=FALSE, "Cool down enabled"=FALSE, "AOL Mode"=enum."Raster", "Plane Mode"=0, "Miniscan Dwell time per pixel (us)"=0.0, "poi dwell time"=0.0, "Number of trials"=0.0, "Number of cycles"=0.0, "Number of pois"=0.0, "Number of miniscans"=0.0, "Number of pixels in miniscan"=0.0, "Rectangle ROI length"=0.0, "Rectangle ROI height"=0.0, "Frame rate (fps)"=0.0, "Acquisition Length"=0.0, "video length (sec)"=0.0, "Stimuli delay (sec)"=0.0, "Cool down time (sec)"=0.0, "Basic Image meta data"={"Wavelength (nm)"=0.0, "# averaged frames"=0.0, "laser power (%)"=0.0, "Pockels"=0.0, "pixel dwell time (us)"=0.0, "pmt 1"=0.0, "pmt 2"=0.0, "back apperture"=0.0, "zoom"=0.0, "field of view"=0.0, "Frame Size"=0, "AOL x centre"=0.0, "AOL y centre"=0.0, "Stage x position"=0.0, "Stage y position"=0.0, "Stage z position"=0.0}, "Z Start (um)"=0.0, "Z Stop (um)"=0.0}, "VOLUME IMAGING"={"Functional Mode"=enum."Point", "Variable Length"=FALSE, "Variable Resolution"=FALSE, "Pockels Modulation"=FALSE, "Stimuli Trigger"=FALSE, "Cool down enabled"=FALSE, "AOL Mode"=enum."Raster", "Plane Mode"=0, "Miniscan Dwell time per pixel (us)"=0.0, "poi dwell time"=0.0, "Number of trials"=0.0, "Number of cycles"=0.0, "Number of pois"=0.0, "Number of miniscans"=0.0, "Number of pixels in miniscan"=0.0, "Rectangle ROI length"=0.0, "Rectangle ROI height"=0.0, "Frame rate (fps)"=0.0, "Acquisition Length"=0.0, "video length (sec)"=0.0, "Stimuli delay (sec)"=0.0, "Cool down time (sec)"=0.0, "Basic Image meta data"={"Wavelength (nm)"=0.0, "# averaged frames"=0.0, "laser power (%)"=0.0, "Pockels"=0.0, "pixel dwell time (us)"=0.0, "pmt 1"=0.0, "pmt 2"=0.0, "back apperture"=0.0, "zoom"=0.0, "field of view"=0.0, "Frame Size"=0, "AOL x centre"=0.0, "AOL y centre"=0.0, "Stage x position"=0.0, "Stage y position"=0.0, "Stage z position"=0.0}, "Z Start (um)"=0.0, "Z Stop (um)"=0.0}, "MOVEMENT CORRECTION"={"Movement Correction"=FALSE, "Axial Reference"=FALSE, "Reference Source"=enum."Green channel", "Full Frame Size"=0.0, "Reference Field of View"=0.0, "Reference Zoom"=0.0, "Reference dwell time (us)"=0.0, "Reference X Pixels"=0.0, "Reference Y Pixels"=0.0, "Number of Z lines"=0.0, "Size of Z pixels"=0.0, "Axial Pixels"=0.0, "Ignore Z lines"=0.0, "Reference Scan Cycles"=0.0, "Reference Threshold XY"=0.0, "Reference Threshold Z"=0.0, "Reference Average XY"=0.0, "Reference Average Z"=0.0, "Proportional Scale"=0.0, "Integral Scale"=0.0, "Proportional Scale Z"=0.0, "Integral Scale Z"=0.0, "Diff Threshold"=0.0, "Diff Threshold Z"=0.0, "Sliding Average"=FALSE, "Reference count reset enabled"=FALSE, "Scan Interval (ms)"=0.0, "Ref Plot Refresh Rate (ms)"=0.0}, "CALIBRATION"={"Pockels Calibration File"=path "", "Calibration_ini file"=path "", "Setup_ini file"=path ""}, "STATISTICS"={"Z-stack duration (sec)"=0.0, "Number of acquired data-points"=0.0, "Acquisition time (ms)"=0.0, "Number of acquired frames"=0.0, "Intertrial times"=[]}, "BIOLOGY INFORMATION"={"Animal Code or Name"="", "Animal DoB"="", "Animal Age"="", "Animal Sex"="", "Animal Weight"="", "Date of Injection"="", "Date of Implant"="", "Site of Injection"="", "Animal Ear Notch"="", "AAV constructs"="", "Genetic background"="", "Optical reporter"="", "Region of brain imaged"="", "Other \ncomments"=""}, "Calibration Data"={"Objective Name"="", "Calibration Wavelength"=0.0, "Sum X"=0.0, "Sum Y"=0.0, "Diff X"=0.0, "Diff Y"=0.0, "Distortion Correction"=0.0, " Z norm to um Scaling"=0.0, " X norm to um Scaling"=0.0}} ("All header parameters in"), "LOGIN"=w14) -> (w13:T6)
    }
    frame "GLOBAL PARAMETERS" {
      n9 = global read "gl_UI Ctrl Refs.vi" "UI ctrl refs"() -> (w26:T27)
      n10 = Unbundle By Name(w26) -> ("Experiment Type"=w25:refnum<vi>)
      n11 = global read "General Globals.vi" "Speed logging enabled"() -> (w29:bool)
      n12 = global read "General Globals.vi" "Microscope Type"() -> (w32:string)
      n13 = global read "General Globals.vi" "Microscope ID"() -> (w33:string)
      n14 = Unbundle By Name(w30) -> ("Field of View (norm)"=w23:dbl, "Fill time (us)"=w22:dbl)
      n15 = global read "General Globals.vi" "Objective"() -> (w31:string)
      n16 = property class="Enum (strict)"(reference=w25) -> ("Value"=w24:T9)  [unwired: 1 in, 2 out]
      n17 = call "fgv_StimTrigLive-Setup.vi"("Function"=enum16{"Intialize", "Write", "Read", "Clear"}."Read") -> ("Live stim.trig.enable"=w27:bool)  [unwired: 11 in, 3 out]
      n18 = Bundle By Name(cluster=T8 {"MicroscopeID"="", "Microscope Type"="", "Objective"="", "Field of View (um)"=0.0, "Fill time (us)"=0.0, "Experiment Type"=enum."In vivo", "Stimuli Trigger"=FALSE, "Speed Logging"=FALSE} ("GLOBAL PARAMETERS"), "MicroscopeID"=w33, "Microscope Type"=w32, "Objective"=w31, "Speed Logging"=w29, "Stimuli Trigger"=w27, "Experiment Type"=w24, "Field of View (um)"=w23, "Fill time (us)"=w22) -> (w21:T8)
      n19 = Bundle By Name(cluster=T6 {"LOGIN"={"User"="", "Profile"="", "Software Version"="", "Experiment Date Time"=timestamp(0 s since 1904-01-01)}, "GLOBAL PARAMETERS"={"MicroscopeID"="", "Microscope Type"="", "Objective"="", "Field of View (um)"=0.0, "Fill time (us)"=0.0, "Experiment Type"=enum."In vivo", "Stimuli Trigger"=FALSE, "Speed Logging"=FALSE}, "IMAGING MODES"={"Time Series"=FALSE, "Motor Zstack"=FALSE, "AOL Zstack"=FALSE, "Functional Imaging"=FALSE, "Volume Imaging"=FALSE}, "TIME SERIES"={"Basic Image meta data"={"Wavelength (nm)"=0.0, "# averaged frames"=0.0, "laser power (%)"=0.0, "Pockels"=0.0, "pixel dwell time (us)"=0.0, "pmt 1"=0.0, "pmt 2"=0.0, "back apperture"=0.0, "zoom"=0.0, "field of view"=0.0, "Frame Size"=0, "AOL x centre"=0.0, "AOL y centre"=0.0, "Stage x position"=0.0, "Stage y position"=0.0, "Stage z position"=0.0}, "AOL z"=0.0}, "MOTOR Z-STACK "={"Hdr Basic Image meta data"={"Wavelength (nm)"=0.0, "# averaged frames"=0.0, "laser power (%)"=0.0, "Pockels"=0.0, "pixel dwell time (us)"=0.0, "pmt 1"=0.0, "pmt 2"=0.0, "back apperture"=0.0, "zoom"=0.0, "field of view"=0.0, "Frame Size"=0, "AOL x centre"=0.0, "AOL y centre"=0.0, "Stage x position"=0.0, "Stage y position"=0.0, "Stage z position"=0.0}, "Z Start"=0.0, "Z Stop"=0.0, "No of Planes"=0, "Laser Power (%) at Z Start"=0.0, "Laser Power (%) at Z Stop"=0.0}, "AOL Z-STACK"={"Hdr Basic Image meta data"={"Wavelength (nm)"=0.0, "# averaged frames"=0.0, "laser power (%)"=0.0, "Pockels"=0.0, "pixel dwell time (us)"=0.0, "pmt 1"=0.0, "pmt 2"=0.0, "back apperture"=0.0, "zoom"=0.0, "field of view"=0.0, "Frame Size"=0, "AOL x centre"=0.0, "AOL y centre"=0.0, "Stage x position"=0.0, "Stage y position"=0.0, "Stage z position"=0.0}, "Z Start"=0.0, "Z Stop"=0.0, "No of Planes"=0, "Laser Power (%) at Z Start"=0.0, "Laser Power (%) at Z Stop"=0.0}, "FUNCTIONAL IMAGING"={"Functional Mode"=enum."Point", "Variable Length"=FALSE, "Variable Resolution"=FALSE, "Pockels Modulation"=FALSE, "Stimuli Trigger"=FALSE, "Cool down enabled"=FALSE, "AOL Mode"=enum."Raster", "Plane Mode"=0, "Miniscan Dwell time per pixel (us)"=0.0, "poi dwell time"=0.0, "Number of trials"=0.0, "Number of cycles"=0.0, "Number of pois"=0.0, "Number of miniscans"=0.0, "Number of pixels in miniscan"=0.0, "Rectangle ROI length"=0.0, "Rectangle ROI height"=0.0, "Frame rate (fps)"=0.0, "Acquisition Length"=0.0, "video length (sec)"=0.0, "Stimuli delay (sec)"=0.0, "Cool down time (sec)"=0.0, "Basic Image meta data"={"Wavelength (nm)"=0.0, "# averaged frames"=0.0, "laser power (%)"=0.0, "Pockels"=0.0, "pixel dwell time (us)"=0.0, "pmt 1"=0.0, "pmt 2"=0.0, "back apperture"=0.0, "zoom"=0.0, "field of view"=0.0, "Frame Size"=0, "AOL x centre"=0.0, "AOL y centre"=0.0, "Stage x position"=0.0, "Stage y position"=0.0, "Stage z position"=0.0}, "Z Start (um)"=0.0, "Z Stop (um)"=0.0}, "VOLUME IMAGING"={"Functional Mode"=enum."Point", "Variable Length"=FALSE, "Variable Resolution"=FALSE, "Pockels Modulation"=FALSE, "Stimuli Trigger"=FALSE, "Cool down enabled"=FALSE, "AOL Mode"=enum."Raster", "Plane Mode"=0, "Miniscan Dwell time per pixel (us)"=0.0, "poi dwell time"=0.0, "Number of trials"=0.0, "Number of cycles"=0.0, "Number of pois"=0.0, "Number of miniscans"=0.0, "Number of pixels in miniscan"=0.0, "Rectangle ROI length"=0.0, "Rectangle ROI height"=0.0, "Frame rate (fps)"=0.0, "Acquisition Length"=0.0, "video length (sec)"=0.0, "Stimuli delay (sec)"=0.0, "Cool down time (sec)"=0.0, "Basic Image meta data"={"Wavelength (nm)"=0.0, "# averaged frames"=0.0, "laser power (%)"=0.0, "Pockels"=0.0, "pixel dwell time (us)"=0.0, "pmt 1"=0.0, "pmt 2"=0.0, "back apperture"=0.0, "zoom"=0.0, "field of view"=0.0, "Frame Size"=0, "AOL x centre"=0.0, "AOL y centre"=0.0, "Stage x position"=0.0, "Stage y position"=0.0, "Stage z position"=0.0}, "Z Start (um)"=0.0, "Z Stop (um)"=0.0}, "MOVEMENT CORRECTION"={"Movement Correction"=FALSE, "Axial Reference"=FALSE, "Reference Source"=enum."Green channel", "Full Frame Size"=0.0, "Reference Field of View"=0.0, "Reference Zoom"=0.0, "Reference dwell time (us)"=0.0, "Reference X Pixels"=0.0, "Reference Y Pixels"=0.0, "Number of Z lines"=0.0, "Size of Z pixels"=0.0, "Axial Pixels"=0.0, "Ignore Z lines"=0.0, "Reference Scan Cycles"=0.0, "Reference Threshold XY"=0.0, "Reference Threshold Z"=0.0, "Reference Average XY"=0.0, "Reference Average Z"=0.0, "Proportional Scale"=0.0, "Integral Scale"=0.0, "Proportional Scale Z"=0.0, "Integral Scale Z"=0.0, "Diff Threshold"=0.0, "Diff Threshold Z"=0.0, "Sliding Average"=FALSE, "Reference count reset enabled"=FALSE, "Scan Interval (ms)"=0.0, "Ref Plot Refresh Rate (ms)"=0.0}, "CALIBRATION"={"Pockels Calibration File"=path "", "Calibration_ini file"=path "", "Setup_ini file"=path ""}, "STATISTICS"={"Z-stack duration (sec)"=0.0, "Number of acquired data-points"=0.0, "Acquisition time (ms)"=0.0, "Number of acquired frames"=0.0, "Intertrial times"=[]}, "BIOLOGY INFORMATION"={"Animal Code or Name"="", "Animal DoB"="", "Animal Age"="", "Animal Sex"="", "Animal Weight"="", "Date of Injection"="", "Date of Implant"="", "Site of Injection"="", "Animal Ear Notch"="", "AAV constructs"="", "Genetic background"="", "Optical reporter"="", "Region of brain imaged"="", "Other \ncomments"=""}, "Calibration Data"={"Objective Name"="", "Calibration Wavelength"=0.0, "Sum X"=0.0, "Sum Y"=0.0, "Diff X"=0.0, "Diff Y"=0.0, "Distortion Correction"=0.0, " Z norm to um Scaling"=0.0, " X norm to um Scaling"=0.0}} ("All header parameters in"), "GLOBAL PARAMETERS"=w21) -> (w20:T6)
    }
    frame "CALIBRATION DATA" {
      n20 = global read "General Globals.vi" "Objective"() -> (w49:string)
      n21 = call "Get norm to um scaling .vi"("Current Objective"=w49) -> ("Objective HW Settings"=w47:T28)  [unwired: 7 in, 3 out]
      n22 = Unbundle By Name(w47) -> ("Name"=w46:string, "Calibrated Wavelength"=w44:dbl, "Sum X"=w45:dbl, "Sum Y"=w43:dbl, "Diff X"=w42:dbl, "Diff Y"=w41:dbl, "Distortion Correction"=w40:dbl, "Z_norm to um_scaling"=w39:dbl, "X_norm to um_scaling"=w38:dbl)
      n23 = Bundle By Name(cluster=T24 {"Objective Name"="", "Calibration Wavelength"=0.0, "Sum X"=0.0, "Sum Y"=0.0, "Diff X"=0.0, "Diff Y"=0.0, "Distortion Correction"=0.0, " Z norm to um Scaling"=0.0, " X norm to um Scaling"=0.0} ("Calibration Data"), "Objective Name"=w46, "Calibration Wavelength"=w44, "Sum X"=w45, "Sum Y"=w43, "Diff X"=w42, "Diff Y"=w41, "Distortion Correction"=w40, "Z norm to um Scaling"=w39, "X norm to um Scaling"=w38) -> (w37:T24)
      n24 = Bundle By Name(cluster=T6 {"LOGIN"={"User"="", "Profile"="", "Software Version"="", "Experiment Date Time"=timestamp(0 s since 1904-01-01)}, "GLOBAL PARAMETERS"={"MicroscopeID"="", "Microscope Type"="", "Objective"="", "Field of View (um)"=0.0, "Fill time (us)"=0.0, "Experiment Type"=enum."In vivo", "Stimuli Trigger"=FALSE, "Speed Logging"=FALSE}, "IMAGING MODES"={"Time Series"=FALSE, "Motor Zstack"=FALSE, "AOL Zstack"=FALSE, "Functional Imaging"=FALSE, "Volume Imaging"=FALSE}, "TIME SERIES"={"Basic Image meta data"={"Wavelength (nm)"=0.0, "# averaged frames"=0.0, "laser power (%)"=0.0, "Pockels"=0.0, "pixel dwell time (us)"=0.0, "pmt 1"=0.0, "pmt 2"=0.0, "back apperture"=0.0, "zoom"=0.0, "field of view"=0.0, "Frame Size"=0, "AOL x centre"=0.0, "AOL y centre"=0.0, "Stage x position"=0.0, "Stage y position"=0.0, "Stage z position"=0.0}, "AOL z"=0.0}, "MOTOR Z-STACK "={"Hdr Basic Image meta data"={"Wavelength (nm)"=0.0, "# averaged frames"=0.0, "laser power (%)"=0.0, "Pockels"=0.0, "pixel dwell time (us)"=0.0, "pmt 1"=0.0, "pmt 2"=0.0, "back apperture"=0.0, "zoom"=0.0, "field of view"=0.0, "Frame Size"=0, "AOL x centre"=0.0, "AOL y centre"=0.0, "Stage x position"=0.0, "Stage y position"=0.0, "Stage z position"=0.0}, "Z Start"=0.0, "Z Stop"=0.0, "No of Planes"=0, "Laser Power (%) at Z Start"=0.0, "Laser Power (%) at Z Stop"=0.0}, "AOL Z-STACK"={"Hdr Basic Image meta data"={"Wavelength (nm)"=0.0, "# averaged frames"=0.0, "laser power (%)"=0.0, "Pockels"=0.0, "pixel dwell time (us)"=0.0, "pmt 1"=0.0, "pmt 2"=0.0, "back apperture"=0.0, "zoom"=0.0, "field of view"=0.0, "Frame Size"=0, "AOL x centre"=0.0, "AOL y centre"=0.0, "Stage x position"=0.0, "Stage y position"=0.0, "Stage z position"=0.0}, "Z Start"=0.0, "Z Stop"=0.0, "No of Planes"=0, "Laser Power (%) at Z Start"=0.0, "Laser Power (%) at Z Stop"=0.0}, "FUNCTIONAL IMAGING"={"Functional Mode"=enum."Point", "Variable Length"=FALSE, "Variable Resolution"=FALSE, "Pockels Modulation"=FALSE, "Stimuli Trigger"=FALSE, "Cool down enabled"=FALSE, "AOL Mode"=enum."Raster", "Plane Mode"=0, "Miniscan Dwell time per pixel (us)"=0.0, "poi dwell time"=0.0, "Number of trials"=0.0, "Number of cycles"=0.0, "Number of pois"=0.0, "Number of miniscans"=0.0, "Number of pixels in miniscan"=0.0, "Rectangle ROI length"=0.0, "Rectangle ROI height"=0.0, "Frame rate (fps)"=0.0, "Acquisition Length"=0.0, "video length (sec)"=0.0, "Stimuli delay (sec)"=0.0, "Cool down time (sec)"=0.0, "Basic Image meta data"={"Wavelength (nm)"=0.0, "# averaged frames"=0.0, "laser power (%)"=0.0, "Pockels"=0.0, "pixel dwell time (us)"=0.0, "pmt 1"=0.0, "pmt 2"=0.0, "back apperture"=0.0, "zoom"=0.0, "field of view"=0.0, "Frame Size"=0, "AOL x centre"=0.0, "AOL y centre"=0.0, "Stage x position"=0.0, "Stage y position"=0.0, "Stage z position"=0.0}, "Z Start (um)"=0.0, "Z Stop (um)"=0.0}, "VOLUME IMAGING"={"Functional Mode"=enum."Point", "Variable Length"=FALSE, "Variable Resolution"=FALSE, "Pockels Modulation"=FALSE, "Stimuli Trigger"=FALSE, "Cool down enabled"=FALSE, "AOL Mode"=enum."Raster", "Plane Mode"=0, "Miniscan Dwell time per pixel (us)"=0.0, "poi dwell time"=0.0, "Number of trials"=0.0, "Number of cycles"=0.0, "Number of pois"=0.0, "Number of miniscans"=0.0, "Number of pixels in miniscan"=0.0, "Rectangle ROI length"=0.0, "Rectangle ROI height"=0.0, "Frame rate (fps)"=0.0, "Acquisition Length"=0.0, "video length (sec)"=0.0, "Stimuli delay (sec)"=0.0, "Cool down time (sec)"=0.0, "Basic Image meta data"={"Wavelength (nm)"=0.0, "# averaged frames"=0.0, "laser power (%)"=0.0, "Pockels"=0.0, "pixel dwell time (us)"=0.0, "pmt 1"=0.0, "pmt 2"=0.0, "back apperture"=0.0, "zoom"=0.0, "field of view"=0.0, "Frame Size"=0, "AOL x centre"=0.0, "AOL y centre"=0.0, "Stage x position"=0.0, "Stage y position"=0.0, "Stage z position"=0.0}, "Z Start (um)"=0.0, "Z Stop (um)"=0.0}, "MOVEMENT CORRECTION"={"Movement Correction"=FALSE, "Axial Reference"=FALSE, "Reference Source"=enum."Green channel", "Full Frame Size"=0.0, "Reference Field of View"=0.0, "Reference Zoom"=0.0, "Reference dwell time (us)"=0.0, "Reference X Pixels"=0.0, "Reference Y Pixels"=0.0, "Number of Z lines"=0.0, "Size of Z pixels"=0.0, "Axial Pixels"=0.0, "Ignore Z lines"=0.0, "Reference Scan Cycles"=0.0, "Reference Threshold XY"=0.0, "Reference Threshold Z"=0.0, "Reference Average XY"=0.0, "Reference Average Z"=0.0, "Proportional Scale"=0.0, "Integral Scale"=0.0, "Proportional Scale Z"=0.0, "Integral Scale Z"=0.0, "Diff Threshold"=0.0, "Diff Threshold Z"=0.0, "Sliding Average"=FALSE, "Reference count reset enabled"=FALSE, "Scan Interval (ms)"=0.0, "Ref Plot Refresh Rate (ms)"=0.0}, "CALIBRATION"={"Pockels Calibration File"=path "", "Calibration_ini file"=path "", "Setup_ini file"=path ""}, "STATISTICS"={"Z-stack duration (sec)"=0.0, "Number of acquired data-points"=0.0, "Acquisition time (ms)"=0.0, "Number of acquired frames"=0.0, "Intertrial times"=[]}, "BIOLOGY INFORMATION"={"Animal Code or Name"="", "Animal DoB"="", "Animal Age"="", "Animal Sex"="", "Animal Weight"="", "Date of Injection"="", "Date of Implant"="", "Site of Injection"="", "Animal Ear Notch"="", "AAV constructs"="", "Genetic background"="", "Optical reporter"="", "Region of brain imaged"="", "Other \ncomments"=""}, "Calibration Data"={"Objective Name"="", "Calibration Wavelength"=0.0, "Sum X"=0.0, "Sum Y"=0.0, "Diff X"=0.0, "Diff Y"=0.0, "Distortion Correction"=0.0, " Z norm to um Scaling"=0.0, " X norm to um Scaling"=0.0}} ("All header parameters in"), "Calibration Data"=w37) -> (w36:T6)
    }
    frame "IMAGING MODES" {
      w51 = FALSE ("Time Series")
      # "This is a place holder case only. The imaging modes will not be updated from here, typically"
      n25 = Bundle By Name(cluster=T10 {"Time Series"=FALSE, "Motor Zstack"=FALSE, "AOL Zstack"=FALSE, "Functional Imaging"=FALSE, "Volume Imaging"=FALSE} ("IMAGING MODES"), "Time Series"=w51, "Motor Zstack"=w51, "AOL Zstack"=w51, "Functional Imaging"=w51, "Volume Imaging"=w51) -> (w53:T10)
      n26 = Bundle By Name(cluster=T6 {"LOGIN"={"User"="", "Profile"="", "Software Version"="", "Experiment Date Time"=timestamp(0 s since 1904-01-01)}, "GLOBAL PARAMETERS"={"MicroscopeID"="", "Microscope Type"="", "Objective"="", "Field of View (um)"=0.0, "Fill time (us)"=0.0, "Experiment Type"=enum."In vivo", "Stimuli Trigger"=FALSE, "Speed Logging"=FALSE}, "IMAGING MODES"={"Time Series"=FALSE, "Motor Zstack"=FALSE, "AOL Zstack"=FALSE, "Functional Imaging"=FALSE, "Volume Imaging"=FALSE}, "TIME SERIES"={"Basic Image meta data"={"Wavelength (nm)"=0.0, "# averaged frames"=0.0, "laser power (%)"=0.0, "Pockels"=0.0, "pixel dwell time (us)"=0.0, "pmt 1"=0.0, "pmt 2"=0.0, "back apperture"=0.0, "zoom"=0.0, "field of view"=0.0, "Frame Size"=0, "AOL x centre"=0.0, "AOL y centre"=0.0, "Stage x position"=0.0, "Stage y position"=0.0, "Stage z position"=0.0}, "AOL z"=0.0}, "MOTOR Z-STACK "={"Hdr Basic Image meta data"={"Wavelength (nm)"=0.0, "# averaged frames"=0.0, "laser power (%)"=0.0, "Pockels"=0.0, "pixel dwell time (us)"=0.0, "pmt 1"=0.0, "pmt 2"=0.0, "back apperture"=0.0, "zoom"=0.0, "field of view"=0.0, "Frame Size"=0, "AOL x centre"=0.0, "AOL y centre"=0.0, "Stage x position"=0.0, "Stage y position"=0.0, "Stage z position"=0.0}, "Z Start"=0.0, "Z Stop"=0.0, "No of Planes"=0, "Laser Power (%) at Z Start"=0.0, "Laser Power (%) at Z Stop"=0.0}, "AOL Z-STACK"={"Hdr Basic Image meta data"={"Wavelength (nm)"=0.0, "# averaged frames"=0.0, "laser power (%)"=0.0, "Pockels"=0.0, "pixel dwell time (us)"=0.0, "pmt 1"=0.0, "pmt 2"=0.0, "back apperture"=0.0, "zoom"=0.0, "field of view"=0.0, "Frame Size"=0, "AOL x centre"=0.0, "AOL y centre"=0.0, "Stage x position"=0.0, "Stage y position"=0.0, "Stage z position"=0.0}, "Z Start"=0.0, "Z Stop"=0.0, "No of Planes"=0, "Laser Power (%) at Z Start"=0.0, "Laser Power (%) at Z Stop"=0.0}, "FUNCTIONAL IMAGING"={"Functional Mode"=enum."Point", "Variable Length"=FALSE, "Variable Resolution"=FALSE, "Pockels Modulation"=FALSE, "Stimuli Trigger"=FALSE, "Cool down enabled"=FALSE, "AOL Mode"=enum."Raster", "Plane Mode"=0, "Miniscan Dwell time per pixel (us)"=0.0, "poi dwell time"=0.0, "Number of trials"=0.0, "Number of cycles"=0.0, "Number of pois"=0.0, "Number of miniscans"=0.0, "Number of pixels in miniscan"=0.0, "Rectangle ROI length"=0.0, "Rectangle ROI height"=0.0, "Frame rate (fps)"=0.0, "Acquisition Length"=0.0, "video length (sec)"=0.0, "Stimuli delay (sec)"=0.0, "Cool down time (sec)"=0.0, "Basic Image meta data"={"Wavelength (nm)"=0.0, "# averaged frames"=0.0, "laser power (%)"=0.0, "Pockels"=0.0, "pixel dwell time (us)"=0.0, "pmt 1"=0.0, "pmt 2"=0.0, "back apperture"=0.0, "zoom"=0.0, "field of view"=0.0, "Frame Size"=0, "AOL x centre"=0.0, "AOL y centre"=0.0, "Stage x position"=0.0, "Stage y position"=0.0, "Stage z position"=0.0}, "Z Start (um)"=0.0, "Z Stop (um)"=0.0}, "VOLUME IMAGING"={"Functional Mode"=enum."Point", "Variable Length"=FALSE, "Variable Resolution"=FALSE, "Pockels Modulation"=FALSE, "Stimuli Trigger"=FALSE, "Cool down enabled"=FALSE, "AOL Mode"=enum."Raster", "Plane Mode"=0, "Miniscan Dwell time per pixel (us)"=0.0, "poi dwell time"=0.0, "Number of trials"=0.0, "Number of cycles"=0.0, "Number of pois"=0.0, "Number of miniscans"=0.0, "Number of pixels in miniscan"=0.0, "Rectangle ROI length"=0.0, "Rectangle ROI height"=0.0, "Frame rate (fps)"=0.0, "Acquisition Length"=0.0, "video length (sec)"=0.0, "Stimuli delay (sec)"=0.0, "Cool down time (sec)"=0.0, "Basic Image meta data"={"Wavelength (nm)"=0.0, "# averaged frames"=0.0, "laser power (%)"=0.0, "Pockels"=0.0, "pixel dwell time (us)"=0.0, "pmt 1"=0.0, "pmt 2"=0.0, "back apperture"=0.0, "zoom"=0.0, "field of view"=0.0, "Frame Size"=0, "AOL x centre"=0.0, "AOL y centre"=0.0, "Stage x position"=0.0, "Stage y position"=0.0, "Stage z position"=0.0}, "Z Start (um)"=0.0, "Z Stop (um)"=0.0}, "MOVEMENT CORRECTION"={"Movement Correction"=FALSE, "Axial Reference"=FALSE, "Reference Source"=enum."Green channel", "Full Frame Size"=0.0, "Reference Field of View"=0.0, "Reference Zoom"=0.0, "Reference dwell time (us)"=0.0, "Reference X Pixels"=0.0, "Reference Y Pixels"=0.0, "Number of Z lines"=0.0, "Size of Z pixels"=0.0, "Axial Pixels"=0.0, "Ignore Z lines"=0.0, "Reference Scan Cycles"=0.0, "Reference Threshold XY"=0.0, "Reference Threshold Z"=0.0, "Reference Average XY"=0.0, "Reference Average Z"=0.0, "Proportional Scale"=0.0, "Integral Scale"=0.0, "Proportional Scale Z"=0.0, "Integral Scale Z"=0.0, "Diff Threshold"=0.0, "Diff Threshold Z"=0.0, "Sliding Average"=FALSE, "Reference count reset enabled"=FALSE, "Scan Interval (ms)"=0.0, "Ref Plot Refresh Rate (ms)"=0.0}, "CALIBRATION"={"Pockels Calibration File"=path "", "Calibration_ini file"=path "", "Setup_ini file"=path ""}, "STATISTICS"={"Z-stack duration (sec)"=0.0, "Number of acquired data-points"=0.0, "Acquisition time (ms)"=0.0, "Number of acquired frames"=0.0, "Intertrial times"=[]}, "BIOLOGY INFORMATION"={"Animal Code or Name"="", "Animal DoB"="", "Animal Age"="", "Animal Sex"="", "Animal Weight"="", "Date of Injection"="", "Date of Implant"="", "Site of Injection"="", "Animal Ear Notch"="", "AAV constructs"="", "Genetic background"="", "Optical reporter"="", "Region of brain imaged"="", "Other \ncomments"=""}, "Calibration Data"={"Objective Name"="", "Calibration Wavelength"=0.0, "Sum X"=0.0, "Sum Y"=0.0, "Diff X"=0.0, "Diff Y"=0.0, "Distortion Correction"=0.0, " Z norm to um Scaling"=0.0, " X norm to um Scaling"=0.0}} ("All header parameters in"), "IMAGING MODES"=w53) -> (w52:T6)
    }
    frame "TIME SERIES" {
      n27 = global read "General Globals.vi" "Timelapse?"() -> (w55:bool)
      n28 = case shown="True" w55 {
        tunnel: [T6 {"LOGIN"={"User"="", "Profile"="", "Software Version"="", "Experiment Date Time"=timestamp(0 s since 1904-01-01)}, "GLOBAL PARAMETERS"={"MicroscopeID"="", "Microscope Type"="", "Objective"="", "Field of View (um)"=0.0, "Fill time (us)"=0.0, "Experiment Type"=enum."In vivo", "Stimuli Trigger"=FALSE, "Speed Logging"=FALSE}, "IMAGING MODES"={"Time Series"=FALSE, "Motor Zstack"=FALSE, "AOL Zstack"=FALSE, "Functional Imaging"=FALSE, "Volume Imaging"=FALSE}, "TIME SERIES"={"Basic Image meta data"={"Wavelength (nm)"=0.0, "# averaged frames"=0.0, "laser power (%)"=0.0, "Pockels"=0.0, "pixel dwell time (us)"=0.0, "pmt 1"=0.0, "pmt 2"=0.0, "back apperture"=0.0, "zoom"=0.0, "field of view"=0.0, "Frame Size"=0, "AOL x centre"=0.0, "AOL y centre"=0.0, "Stage x position"=0.0, "Stage y position"=0.0, "Stage z position"=0.0}, "AOL z"=0.0}, "MOTOR Z-STACK "={"Hdr Basic Image meta data"={"Wavelength (nm)"=0.0, "# averaged frames"=0.0, "laser power (%)"=0.0, "Pockels"=0.0, "pixel dwell time (us)"=0.0, "pmt 1"=0.0, "pmt 2"=0.0, "back apperture"=0.0, "zoom"=0.0, "field of view"=0.0, "Frame Size"=0, "AOL x centre"=0.0, "AOL y centre"=0.0, "Stage x position"=0.0, "Stage y position"=0.0, "Stage z position"=0.0}, "Z Start"=0.0, "Z Stop"=0.0, "No of Planes"=0, "Laser Power (%) at Z Start"=0.0, "Laser Power (%) at Z Stop"=0.0}, "AOL Z-STACK"={"Hdr Basic Image meta data"={"Wavelength (nm)"=0.0, "# averaged frames"=0.0, "laser power (%)"=0.0, "Pockels"=0.0, "pixel dwell time (us)"=0.0, "pmt 1"=0.0, "pmt 2"=0.0, "back apperture"=0.0, "zoom"=0.0, "field of view"=0.0, "Frame Size"=0, "AOL x centre"=0.0, "AOL y centre"=0.0, "Stage x position"=0.0, "Stage y position"=0.0, "Stage z position"=0.0}, "Z Start"=0.0, "Z Stop"=0.0, "No of Planes"=0, "Laser Power (%) at Z Start"=0.0, "Laser Power (%) at Z Stop"=0.0}, "FUNCTIONAL IMAGING"={"Functional Mode"=enum."Point", "Variable Length"=FALSE, "Variable Resolution"=FALSE, "Pockels Modulation"=FALSE, "Stimuli Trigger"=FALSE, "Cool down enabled"=FALSE, "AOL Mode"=enum."Raster", "Plane Mode"=0, "Miniscan Dwell time per pixel (us)"=0.0, "poi dwell time"=0.0, "Number of trials"=0.0, "Number of cycles"=0.0, "Number of pois"=0.0, "Number of miniscans"=0.0, "Number of pixels in miniscan"=0.0, "Rectangle ROI length"=0.0, "Rectangle ROI height"=0.0, "Frame rate (fps)"=0.0, "Acquisition Length"=0.0, "video length (sec)"=0.0, "Stimuli delay (sec)"=0.0, "Cool down time (sec)"=0.0, "Basic Image meta data"={"Wavelength (nm)"=0.0, "# averaged frames"=0.0, "laser power (%)"=0.0, "Pockels"=0.0, "pixel dwell time (us)"=0.0, "pmt 1"=0.0, "pmt 2"=0.0, "back apperture"=0.0, "zoom"=0.0, "field of view"=0.0, "Frame Size"=0, "AOL x centre"=0.0, "AOL y centre"=0.0, "Stage x position"=0.0, "Stage y position"=0.0, "Stage z position"=0.0}, "Z Start (um)"=0.0, "Z Stop (um)"=0.0}, "VOLUME IMAGING"={"Functional Mode"=enum."Point", "Variable Length"=FALSE, "Variable Resolution"=FALSE, "Pockels Modulation"=FALSE, "Stimuli Trigger"=FALSE, "Cool down enabled"=FALSE, "AOL Mode"=enum."Raster", "Plane Mode"=0, "Miniscan Dwell time per pixel (us)"=0.0, "poi dwell time"=0.0, "Number of trials"=0.0, "Number of cycles"=0.0, "Number of pois"=0.0, "Number of miniscans"=0.0, "Number of pixels in miniscan"=0.0, "Rectangle ROI length"=0.0, "Rectangle ROI height"=0.0, "Frame rate (fps)"=0.0, "Acquisition Length"=0.0, "video length (sec)"=0.0, "Stimuli delay (sec)"=0.0, "Cool down time (sec)"=0.0, "Basic Image meta data"={"Wavelength (nm)"=0.0, "# averaged frames"=0.0, "laser power (%)"=0.0, "Pockels"=0.0, "pixel dwell time (us)"=0.0, "pmt 1"=0.0, "pmt 2"=0.0, "back apperture"=0.0, "zoom"=0.0, "field of view"=0.0, "Frame Size"=0, "AOL x centre"=0.0, "AOL y centre"=0.0, "Stage x position"=0.0, "Stage y position"=0.0, "Stage z position"=0.0}, "Z Start (um)"=0.0, "Z Stop (um)"=0.0}, "MOVEMENT CORRECTION"={"Movement Correction"=FALSE, "Axial Reference"=FALSE, "Reference Source"=enum."Green channel", "Full Frame Size"=0.0, "Reference Field of View"=0.0, "Reference Zoom"=0.0, "Reference dwell time (us)"=0.0, "Reference X Pixels"=0.0, "Reference Y Pixels"=0.0, "Number of Z lines"=0.0, "Size of Z pixels"=0.0, "Axial Pixels"=0.0, "Ignore Z lines"=0.0, "Reference Scan Cycles"=0.0, "Reference Threshold XY"=0.0, "Reference Threshold Z"=0.0, "Reference Average XY"=0.0, "Reference Average Z"=0.0, "Proportional Scale"=0.0, "Integral Scale"=0.0, "Proportional Scale Z"=0.0, "Integral Scale Z"=0.0, "Diff Threshold"=0.0, "Diff Threshold Z"=0.0, "Sliding Average"=FALSE, "Reference count reset enabled"=FALSE, "Scan Interval (ms)"=0.0, "Ref Plot Refresh Rate (ms)"=0.0}, "CALIBRATION"={"Pockels Calibration File"=path "", "Calibration_ini file"=path "", "Setup_ini file"=path ""}, "STATISTICS"={"Z-stack duration (sec)"=0.0, "Number of acquired data-points"=0.0, "Acquisition time (ms)"=0.0, "Number of acquired frames"=0.0, "Intertrial times"=[]}, "BIOLOGY INFORMATION"={"Animal Code or Name"="", "Animal DoB"="", "Animal Age"="", "Animal Sex"="", "Animal Weight"="", "Date of Injection"="", "Date of Implant"="", "Site of Injection"="", "Animal Ear Notch"="", "AAV constructs"="", "Genetic background"="", "Optical reporter"="", "Region of brain imaged"="", "Other \ncomments"=""}, "Calibration Data"={"Objective Name"="", "Calibration Wavelength"=0.0, "Sum X"=0.0, "Sum Y"=0.0, "Diff X"=0.0, "Diff Y"=0.0, "Distortion Correction"=0.0, " Z norm to um Scaling"=0.0, " X norm to um Scaling"=0.0}} ("All header parameters in") w62] -> w57
        tunnel: w56 -> [_ w61]
        frame False {
        }
        frame True {
          n29 = call "Experiment header-bundle basic image meta data.vi"("AOL_Globals"=w61) -> ("Basic image meta-data"=w65:T12)  [unwired: 10 in]
          n30 = Unbundle By Name(w61) -> ("AOL Z"=w60:dbl)
          n31 = Bundle By Name(cluster=T11 {"Basic Image meta data"={"Wavelength (nm)"=0.0, "# averaged frames"=0.0, "laser power (%)"=0.0, "Pockels"=0.0, "pixel dwell time (us)"=0.0, "pmt 1"=0.0, "pmt 2"=0.0, "back apperture"=0.0, "zoom"=0.0, "field of view"=0.0, "Frame Size"=0, "AOL x centre"=0.0, "AOL y centre"=0.0, "Stage x position"=0.0, "Stage y position"=0.0, "Stage z position"=0.0}, "AOL z"=0.0} ("TIME SERIES"), "Basic Image meta data"=w65, "AOL z"=w60) -> (w63:T11)
          n32 = Bundle By Name(cluster=T6 {"LOGIN"={"User"="", "Profile"="", "Software Version"="", "Experiment Date Time"=timestamp(0 s since 1904-01-01)}, "GLOBAL PARAMETERS"={"MicroscopeID"="", "Microscope Type"="", "Objective"="", "Field of View (um)"=0.0, "Fill time (us)"=0.0, "Experiment Type"=enum."In vivo", "Stimuli Trigger"=FALSE, "Speed Logging"=FALSE}, "IMAGING MODES"={"Time Series"=FALSE, "Motor Zstack"=FALSE, "AOL Zstack"=FALSE, "Functional Imaging"=FALSE, "Volume Imaging"=FALSE}, "TIME SERIES"={"Basic Image meta data"={"Wavelength (nm)"=0.0, "# averaged frames"=0.0, "laser power (%)"=0.0, "Pockels"=0.0, "pixel dwell time (us)"=0.0, "pmt 1"=0.0, "pmt 2"=0.0, "back apperture"=0.0, "zoom"=0.0, "field of view"=0.0, "Frame Size"=0, "AOL x centre"=0.0, "AOL y centre"=0.0, "Stage x position"=0.0, "Stage y position"=0.0, "Stage z position"=0.0}, "AOL z"=0.0}, "MOTOR Z-STACK "={"Hdr Basic Image meta data"={"Wavelength (nm)"=0.0, "# averaged frames"=0.0, "laser power (%)"=0.0, "Pockels"=0.0, "pixel dwell time (us)"=0.0, "pmt 1"=0.0, "pmt 2"=0.0, "back apperture"=0.0, "zoom"=0.0, "field of view"=0.0, "Frame Size"=0, "AOL x centre"=0.0, "AOL y centre"=0.0, "Stage x position"=0.0, "Stage y position"=0.0, "Stage z position"=0.0}, "Z Start"=0.0, "Z Stop"=0.0, "No of Planes"=0, "Laser Power (%) at Z Start"=0.0, "Laser Power (%) at Z Stop"=0.0}, "AOL Z-STACK"={"Hdr Basic Image meta data"={"Wavelength (nm)"=0.0, "# averaged frames"=0.0, "laser power (%)"=0.0, "Pockels"=0.0, "pixel dwell time (us)"=0.0, "pmt 1"=0.0, "pmt 2"=0.0, "back apperture"=0.0, "zoom"=0.0, "field of view"=0.0, "Frame Size"=0, "AOL x centre"=0.0, "AOL y centre"=0.0, "Stage x position"=0.0, "Stage y position"=0.0, "Stage z position"=0.0}, "Z Start"=0.0, "Z Stop"=0.0, "No of Planes"=0, "Laser Power (%) at Z Start"=0.0, "Laser Power (%) at Z Stop"=0.0}, "FUNCTIONAL IMAGING"={"Functional Mode"=enum."Point", "Variable Length"=FALSE, "Variable Resolution"=FALSE, "Pockels Modulation"=FALSE, "Stimuli Trigger"=FALSE, "Cool down enabled"=FALSE, "AOL Mode"=enum."Raster", "Plane Mode"=0, "Miniscan Dwell time per pixel (us)"=0.0, "poi dwell time"=0.0, "Number of trials"=0.0, "Number of cycles"=0.0, "Number of pois"=0.0, "Number of miniscans"=0.0, "Number of pixels in miniscan"=0.0, "Rectangle ROI length"=0.0, "Rectangle ROI height"=0.0, "Frame rate (fps)"=0.0, "Acquisition Length"=0.0, "video length (sec)"=0.0, "Stimuli delay (sec)"=0.0, "Cool down time (sec)"=0.0, "Basic Image meta data"={"Wavelength (nm)"=0.0, "# averaged frames"=0.0, "laser power (%)"=0.0, "Pockels"=0.0, "pixel dwell time (us)"=0.0, "pmt 1"=0.0, "pmt 2"=0.0, "back apperture"=0.0, "zoom"=0.0, "field of view"=0.0, "Frame Size"=0, "AOL x centre"=0.0, "AOL y centre"=0.0, "Stage x position"=0.0, "Stage y position"=0.0, "Stage z position"=0.0}, "Z Start (um)"=0.0, "Z Stop (um)"=0.0}, "VOLUME IMAGING"={"Functional Mode"=enum."Point", "Variable Length"=FALSE, "Variable Resolution"=FALSE, "Pockels Modulation"=FALSE, "Stimuli Trigger"=FALSE, "Cool down enabled"=FALSE, "AOL Mode"=enum."Raster", "Plane Mode"=0, "Miniscan Dwell time per pixel (us)"=0.0, "poi dwell time"=0.0, "Number of trials"=0.0, "Number of cycles"=0.0, "Number of pois"=0.0, "Number of miniscans"=0.0, "Number of pixels in miniscan"=0.0, "Rectangle ROI length"=0.0, "Rectangle ROI height"=0.0, "Frame rate (fps)"=0.0, "Acquisition Length"=0.0, "video length (sec)"=0.0, "Stimuli delay (sec)"=0.0, "Cool down time (sec)"=0.0, "Basic Image meta data"={"Wavelength (nm)"=0.0, "# averaged frames"=0.0, "laser power (%)"=0.0, "Pockels"=0.0, "pixel dwell time (us)"=0.0, "pmt 1"=0.0, "pmt 2"=0.0, "back apperture"=0.0, "zoom"=0.0, "field of view"=0.0, "Frame Size"=0, "AOL x centre"=0.0, "AOL y centre"=0.0, "Stage x position"=0.0, "Stage y position"=0.0, "Stage z position"=0.0}, "Z Start (um)"=0.0, "Z Stop (um)"=0.0}, "MOVEMENT CORRECTION"={"Movement Correction"=FALSE, "Axial Reference"=FALSE, "Reference Source"=enum."Green channel", "Full Frame Size"=0.0, "Reference Field of View"=0.0, "Reference Zoom"=0.0, "Reference dwell time (us)"=0.0, "Reference X Pixels"=0.0, "Reference Y Pixels"=0.0, "Number of Z lines"=0.0, "Size of Z pixels"=0.0, "Axial Pixels"=0.0, "Ignore Z lines"=0.0, "Reference Scan Cycles"=0.0, "Reference Threshold XY"=0.0, "Reference Threshold Z"=0.0, "Reference Average XY"=0.0, "Reference Average Z"=0.0, "Proportional Scale"=0.0, "Integral Scale"=0.0, "Proportional Scale Z"=0.0, "Integral Scale Z"=0.0, "Diff Threshold"=0.0, "Diff Threshold Z"=0.0, "Sliding Average"=FALSE, "Reference count reset enabled"=FALSE, "Scan Interval (ms)"=0.0, "Ref Plot Refresh Rate (ms)"=0.0}, "CALIBRATION"={"Pockels Calibration File"=path "", "Calibration_ini file"=path "", "Setup_ini file"=path ""}, "STATISTICS"={"Z-stack duration (sec)"=0.0, "Number of acquired data-points"=0.0, "Acquisition time (ms)"=0.0, "Number of acquired frames"=0.0, "Intertrial times"=[]}, "BIOLOGY INFORMATION"={"Animal Code or Name"="", "Animal DoB"="", "Animal Age"="", "Animal Sex"="", "Animal Weight"="", "Date of Injection"="", "Date of Implant"="", "Site of Injection"="", "Animal Ear Notch"="", "AAV constructs"="", "Genetic background"="", "Optical reporter"="", "Region of brain imaged"="", "Other \ncomments"=""}, "Calibration Data"={"Objective Name"="", "Calibration Wavelength"=0.0, "Sum X"=0.0, "Sum Y"=0.0, "Diff X"=0.0, "Diff Y"=0.0, "Distortion Correction"=0.0, " Z norm to um Scaling"=0.0, " X norm to um Scaling"=0.0}} ("All header parameters in"), "TIME SERIES"=w63) -> (w62:T6)
        }
      }
    }
    frame "MOTOR Z-STACK" {
      n33 = Unbundle By Name(w72) -> ("Z Start"=w70:dbl, "Z Stop"=w69:dbl, "# Planes"=w71:i32, "Laser power (%) at Z Start"=w68:u8, "Laser power (%) at Z Stop"=w67:u8)
      n34 = call "Experiment header-bundle basic image meta data.vi"("AOL_Globals"=w72) -> ("Basic image meta-data"=w76:T12)  [unwired: 10 in]
      n35 = Bundle By Name(cluster=T13 {"Hdr Basic Image meta data"={"Wavelength (nm)"=0.0, "# averaged frames"=0.0, "laser power (%)"=0.0, "Pockels"=0.0, "pixel dwell time (us)"=0.0, "pmt 1"=0.0, "pmt 2"=0.0, "back apperture"=0.0, "zoom"=0.0, "field of view"=0.0, "Frame Size"=0, "AOL x centre"=0.0, "AOL y centre"=0.0, "Stage x position"=0.0, "Stage y position"=0.0, "Stage z position"=0.0}, "Z Start"=0.0, "Z Stop"=0.0, "No of Planes"=0, "Laser Power (%) at Z Start"=0.0, "Laser Power (%) at Z Stop"=0.0} ("MOTOR Z-STACK"), "Hdr Basic Image meta data"=w76, "Z Start"=w70, "Z Stop"=w69, "No of Planes"=w71, "Laser Power (%) at Z Start"=w68, "Laser Power (%) at Z Stop"=w67) -> (w74:T13)
      n36 = Bundle By Name(cluster=T6 {"LOGIN"={"User"="", "Profile"="", "Software Version"="", "Experiment Date Time"=timestamp(0 s since 1904-01-01)}, "GLOBAL PARAMETERS"={"MicroscopeID"="", "Microscope Type"="", "Objective"="", "Field of View (um)"=0.0, "Fill time (us)"=0.0, "Experiment Type"=enum."In vivo", "Stimuli Trigger"=FALSE, "Speed Logging"=FALSE}, "IMAGING MODES"={"Time Series"=FALSE, "Motor Zstack"=FALSE, "AOL Zstack"=FALSE, "Functional Imaging"=FALSE, "Volume Imaging"=FALSE}, "TIME SERIES"={"Basic Image meta data"={"Wavelength (nm)"=0.0, "# averaged frames"=0.0, "laser power (%)"=0.0, "Pockels"=0.0, "pixel dwell time (us)"=0.0, "pmt 1"=0.0, "pmt 2"=0.0, "back apperture"=0.0, "zoom"=0.0, "field of view"=0.0, "Frame Size"=0, "AOL x centre"=0.0, "AOL y centre"=0.0, "Stage x position"=0.0, "Stage y position"=0.0, "Stage z position"=0.0}, "AOL z"=0.0}, "MOTOR Z-STACK "={"Hdr Basic Image meta data"={"Wavelength (nm)"=0.0, "# averaged frames"=0.0, "laser power (%)"=0.0, "Pockels"=0.0, "pixel dwell time (us)"=0.0, "pmt 1"=0.0, "pmt 2"=0.0, "back apperture"=0.0, "zoom"=0.0, "field of view"=0.0, "Frame Size"=0, "AOL x centre"=0.0, "AOL y centre"=0.0, "Stage x position"=0.0, "Stage y position"=0.0, "Stage z position"=0.0}, "Z Start"=0.0, "Z Stop"=0.0, "No of Planes"=0, "Laser Power (%) at Z Start"=0.0, "Laser Power (%) at Z Stop"=0.0}, "AOL Z-STACK"={"Hdr Basic Image meta data"={"Wavelength (nm)"=0.0, "# averaged frames"=0.0, "laser power (%)"=0.0, "Pockels"=0.0, "pixel dwell time (us)"=0.0, "pmt 1"=0.0, "pmt 2"=0.0, "back apperture"=0.0, "zoom"=0.0, "field of view"=0.0, "Frame Size"=0, "AOL x centre"=0.0, "AOL y centre"=0.0, "Stage x position"=0.0, "Stage y position"=0.0, "Stage z position"=0.0}, "Z Start"=0.0, "Z Stop"=0.0, "No of Planes"=0, "Laser Power (%) at Z Start"=0.0, "Laser Power (%) at Z Stop"=0.0}, "FUNCTIONAL IMAGING"={"Functional Mode"=enum."Point", "Variable Length"=FALSE, "Variable Resolution"=FALSE, "Pockels Modulation"=FALSE, "Stimuli Trigger"=FALSE, "Cool down enabled"=FALSE, "AOL Mode"=enum."Raster", "Plane Mode"=0, "Miniscan Dwell time per pixel (us)"=0.0, "poi dwell time"=0.0, "Number of trials"=0.0, "Number of cycles"=0.0, "Number of pois"=0.0, "Number of miniscans"=0.0, "Number of pixels in miniscan"=0.0, "Rectangle ROI length"=0.0, "Rectangle ROI height"=0.0, "Frame rate (fps)"=0.0, "Acquisition Length"=0.0, "video length (sec)"=0.0, "Stimuli delay (sec)"=0.0, "Cool down time (sec)"=0.0, "Basic Image meta data"={"Wavelength (nm)"=0.0, "# averaged frames"=0.0, "laser power (%)"=0.0, "Pockels"=0.0, "pixel dwell time (us)"=0.0, "pmt 1"=0.0, "pmt 2"=0.0, "back apperture"=0.0, "zoom"=0.0, "field of view"=0.0, "Frame Size"=0, "AOL x centre"=0.0, "AOL y centre"=0.0, "Stage x position"=0.0, "Stage y position"=0.0, "Stage z position"=0.0}, "Z Start (um)"=0.0, "Z Stop (um)"=0.0}, "VOLUME IMAGING"={"Functional Mode"=enum."Point", "Variable Length"=FALSE, "Variable Resolution"=FALSE, "Pockels Modulation"=FALSE, "Stimuli Trigger"=FALSE, "Cool down enabled"=FALSE, "AOL Mode"=enum."Raster", "Plane Mode"=0, "Miniscan Dwell time per pixel (us)"=0.0, "poi dwell time"=0.0, "Number of trials"=0.0, "Number of cycles"=0.0, "Number of pois"=0.0, "Number of miniscans"=0.0, "Number of pixels in miniscan"=0.0, "Rectangle ROI length"=0.0, "Rectangle ROI height"=0.0, "Frame rate (fps)"=0.0, "Acquisition Length"=0.0, "video length (sec)"=0.0, "Stimuli delay (sec)"=0.0, "Cool down time (sec)"=0.0, "Basic Image meta data"={"Wavelength (nm)"=0.0, "# averaged frames"=0.0, "laser power (%)"=0.0, "Pockels"=0.0, "pixel dwell time (us)"=0.0, "pmt 1"=0.0, "pmt 2"=0.0, "back apperture"=0.0, "zoom"=0.0, "field of view"=0.0, "Frame Size"=0, "AOL x centre"=0.0, "AOL y centre"=0.0, "Stage x position"=0.0, "Stage y position"=0.0, "Stage z position"=0.0}, "Z Start (um)"=0.0, "Z Stop (um)"=0.0}, "MOVEMENT CORRECTION"={"Movement Correction"=FALSE, "Axial Reference"=FALSE, "Reference Source"=enum."Green channel", "Full Frame Size"=0.0, "Reference Field of View"=0.0, "Reference Zoom"=0.0, "Reference dwell time (us)"=0.0, "Reference X Pixels"=0.0, "Reference Y Pixels"=0.0, "Number of Z lines"=0.0, "Size of Z pixels"=0.0, "Axial Pixels"=0.0, "Ignore Z lines"=0.0, "Reference Scan Cycles"=0.0, "Reference Threshold XY"=0.0, "Reference Threshold Z"=0.0, "Reference Average XY"=0.0, "Reference Average Z"=0.0, "Proportional Scale"=0.0, "Integral Scale"=0.0, "Proportional Scale Z"=0.0, "Integral Scale Z"=0.0, "Diff Threshold"=0.0, "Diff Threshold Z"=0.0, "Sliding Average"=FALSE, "Reference count reset enabled"=FALSE, "Scan Interval (ms)"=0.0, "Ref Plot Refresh Rate (ms)"=0.0}, "CALIBRATION"={"Pockels Calibration File"=path "", "Calibration_ini file"=path "", "Setup_ini file"=path ""}, "STATISTICS"={"Z-stack duration (sec)"=0.0, "Number of acquired data-points"=0.0, "Acquisition time (ms)"=0.0, "Number of acquired frames"=0.0, "Intertrial times"=[]}, "BIOLOGY INFORMATION"={"Animal Code or Name"="", "Animal DoB"="", "Animal Age"="", "Animal Sex"="", "Animal Weight"="", "Date of Injection"="", "Date of Implant"="", "Site of Injection"="", "Animal Ear Notch"="", "AAV constructs"="", "Genetic background"="", "Optical reporter"="", "Region of brain imaged"="", "Other \ncomments"=""}, "Calibration Data"={"Objective Name"="", "Calibration Wavelength"=0.0, "Sum X"=0.0, "Sum Y"=0.0, "Diff X"=0.0, "Diff Y"=0.0, "Distortion Correction"=0.0, " Z norm to um Scaling"=0.0, " X norm to um Scaling"=0.0}} ("All header parameters in"), "MOTOR Z-STACK"=w74) -> (w73:T6)
    }
    frame "AOL Z-STACK" {
      n37 = Unbundle By Name(w83) -> ("Z Start"=w82:dbl, "Z Stop"=w81:dbl, "# Planes"=w80:i32, "Laser power (%) at Z Start"=w79:u8, "Laser power (%) at Z Stop"=w78:u8)
      n38 = call "Experiment header-bundle basic image meta data.vi"("AOL_Globals"=w83) -> ("Basic image meta-data"=w87:T12)  [unwired: 10 in]
      n39 = Bundle By Name(cluster=T14 {"Hdr Basic Image meta data"={"Wavelength (nm)"=0.0, "# averaged frames"=0.0, "laser power (%)"=0.0, "Pockels"=0.0, "pixel dwell time (us)"=0.0, "pmt 1"=0.0, "pmt 2"=0.0, "back apperture"=0.0, "zoom"=0.0, "field of view"=0.0, "Frame Size"=0, "AOL x centre"=0.0, "AOL y centre"=0.0, "Stage x position"=0.0, "Stage y position"=0.0, "Stage z position"=0.0}, "Z Start"=0.0, "Z Stop"=0.0, "No of Planes"=0, "Laser Power (%) at Z Start"=0.0, "Laser Power (%) at Z Stop"=0.0} ("AOL Z-STACK"), "Hdr Basic Image meta data"=w87, "Z Start"=w82, "Z Stop"=w81, "No of Planes"=w80, "Laser Power (%) at Z Start"=w79, "Laser Power (%) at Z Stop"=w78) -> (w86:T14)
      n40 = Bundle By Name(cluster=T6 {"LOGIN"={"User"="", "Profile"="", "Software Version"="", "Experiment Date Time"=timestamp(0 s since 1904-01-01)}, "GLOBAL PARAMETERS"={"MicroscopeID"="", "Microscope Type"="", "Objective"="", "Field of View (um)"=0.0, "Fill time (us)"=0.0, "Experiment Type"=enum."In vivo", "Stimuli Trigger"=FALSE, "Speed Logging"=FALSE}, "IMAGING MODES"={"Time Series"=FALSE, "Motor Zstack"=FALSE, "AOL Zstack"=FALSE, "Functional Imaging"=FALSE, "Volume Imaging"=FALSE}, "TIME SERIES"={"Basic Image meta data"={"Wavelength (nm)"=0.0, "# averaged frames"=0.0, "laser power (%)"=0.0, "Pockels"=0.0, "pixel dwell time (us)"=0.0, "pmt 1"=0.0, "pmt 2"=0.0, "back apperture"=0.0, "zoom"=0.0, "field of view"=0.0, "Frame Size"=0, "AOL x centre"=0.0, "AOL y centre"=0.0, "Stage x position"=0.0, "Stage y position"=0.0, "Stage z position"=0.0}, "AOL z"=0.0}, "MOTOR Z-STACK "={"Hdr Basic Image meta data"={"Wavelength (nm)"=0.0, "# averaged frames"=0.0, "laser power (%)"=0.0, "Pockels"=0.0, "pixel dwell time (us)"=0.0, "pmt 1"=0.0, "pmt 2"=0.0, "back apperture"=0.0, "zoom"=0.0, "field of view"=0.0, "Frame Size"=0, "AOL x centre"=0.0, "AOL y centre"=0.0, "Stage x position"=0.0, "Stage y position"=0.0, "Stage z position"=0.0}, "Z Start"=0.0, "Z Stop"=0.0, "No of Planes"=0, "Laser Power (%) at Z Start"=0.0, "Laser Power (%) at Z Stop"=0.0}, "AOL Z-STACK"={"Hdr Basic Image meta data"={"Wavelength (nm)"=0.0, "# averaged frames"=0.0, "laser power (%)"=0.0, "Pockels"=0.0, "pixel dwell time (us)"=0.0, "pmt 1"=0.0, "pmt 2"=0.0, "back apperture"=0.0, "zoom"=0.0, "field of view"=0.0, "Frame Size"=0, "AOL x centre"=0.0, "AOL y centre"=0.0, "Stage x position"=0.0, "Stage y position"=0.0, "Stage z position"=0.0}, "Z Start"=0.0, "Z Stop"=0.0, "No of Planes"=0, "Laser Power (%) at Z Start"=0.0, "Laser Power (%) at Z Stop"=0.0}, "FUNCTIONAL IMAGING"={"Functional Mode"=enum."Point", "Variable Length"=FALSE, "Variable Resolution"=FALSE, "Pockels Modulation"=FALSE, "Stimuli Trigger"=FALSE, "Cool down enabled"=FALSE, "AOL Mode"=enum."Raster", "Plane Mode"=0, "Miniscan Dwell time per pixel (us)"=0.0, "poi dwell time"=0.0, "Number of trials"=0.0, "Number of cycles"=0.0, "Number of pois"=0.0, "Number of miniscans"=0.0, "Number of pixels in miniscan"=0.0, "Rectangle ROI length"=0.0, "Rectangle ROI height"=0.0, "Frame rate (fps)"=0.0, "Acquisition Length"=0.0, "video length (sec)"=0.0, "Stimuli delay (sec)"=0.0, "Cool down time (sec)"=0.0, "Basic Image meta data"={"Wavelength (nm)"=0.0, "# averaged frames"=0.0, "laser power (%)"=0.0, "Pockels"=0.0, "pixel dwell time (us)"=0.0, "pmt 1"=0.0, "pmt 2"=0.0, "back apperture"=0.0, "zoom"=0.0, "field of view"=0.0, "Frame Size"=0, "AOL x centre"=0.0, "AOL y centre"=0.0, "Stage x position"=0.0, "Stage y position"=0.0, "Stage z position"=0.0}, "Z Start (um)"=0.0, "Z Stop (um)"=0.0}, "VOLUME IMAGING"={"Functional Mode"=enum."Point", "Variable Length"=FALSE, "Variable Resolution"=FALSE, "Pockels Modulation"=FALSE, "Stimuli Trigger"=FALSE, "Cool down enabled"=FALSE, "AOL Mode"=enum."Raster", "Plane Mode"=0, "Miniscan Dwell time per pixel (us)"=0.0, "poi dwell time"=0.0, "Number of trials"=0.0, "Number of cycles"=0.0, "Number of pois"=0.0, "Number of miniscans"=0.0, "Number of pixels in miniscan"=0.0, "Rectangle ROI length"=0.0, "Rectangle ROI height"=0.0, "Frame rate (fps)"=0.0, "Acquisition Length"=0.0, "video length (sec)"=0.0, "Stimuli delay (sec)"=0.0, "Cool down time (sec)"=0.0, "Basic Image meta data"={"Wavelength (nm)"=0.0, "# averaged frames"=0.0, "laser power (%)"=0.0, "Pockels"=0.0, "pixel dwell time (us)"=0.0, "pmt 1"=0.0, "pmt 2"=0.0, "back apperture"=0.0, "zoom"=0.0, "field of view"=0.0, "Frame Size"=0, "AOL x centre"=0.0, "AOL y centre"=0.0, "Stage x position"=0.0, "Stage y position"=0.0, "Stage z position"=0.0}, "Z Start (um)"=0.0, "Z Stop (um)"=0.0}, "MOVEMENT CORRECTION"={"Movement Correction"=FALSE, "Axial Reference"=FALSE, "Reference Source"=enum."Green channel", "Full Frame Size"=0.0, "Reference Field of View"=0.0, "Reference Zoom"=0.0, "Reference dwell time (us)"=0.0, "Reference X Pixels"=0.0, "Reference Y Pixels"=0.0, "Number of Z lines"=0.0, "Size of Z pixels"=0.0, "Axial Pixels"=0.0, "Ignore Z lines"=0.0, "Reference Scan Cycles"=0.0, "Reference Threshold XY"=0.0, "Reference Threshold Z"=0.0, "Reference Average XY"=0.0, "Reference Average Z"=0.0, "Proportional Scale"=0.0, "Integral Scale"=0.0, "Proportional Scale Z"=0.0, "Integral Scale Z"=0.0, "Diff Threshold"=0.0, "Diff Threshold Z"=0.0, "Sliding Average"=FALSE, "Reference count reset enabled"=FALSE, "Scan Interval (ms)"=0.0, "Ref Plot Refresh Rate (ms)"=0.0}, "CALIBRATION"={"Pockels Calibration File"=path "", "Calibration_ini file"=path "", "Setup_ini file"=path ""}, "STATISTICS"={"Z-stack duration (sec)"=0.0, "Number of acquired data-points"=0.0, "Acquisition time (ms)"=0.0, "Number of acquired frames"=0.0, "Intertrial times"=[]}, "BIOLOGY INFORMATION"={"Animal Code or Name"="", "Animal DoB"="", "Animal Age"="", "Animal Sex"="", "Animal Weight"="", "Date of Injection"="", "Date of Implant"="", "Site of Injection"="", "Animal Ear Notch"="", "AAV constructs"="", "Genetic background"="", "Optical reporter"="", "Region of brain imaged"="", "Other \ncomments"=""}, "Calibration Data"={"Objective Name"="", "Calibration Wavelength"=0.0, "Sum X"=0.0, "Sum Y"=0.0, "Diff X"=0.0, "Diff Y"=0.0, "Distortion Correction"=0.0, " Z norm to um Scaling"=0.0, " X norm to um Scaling"=0.0}} ("All header parameters in"), "AOL Z-STACK"=w86) -> (w85:T6)
    }
    frame "FUNCTIONAL IMAGING" {
      n41 = Unbundle By Name(w99) -> ("Use Variable Length"=w98:bool, "Use Variable Resolution"=w94:bool)
      n42 = call "fgv_Cool down setup.vi"("Function"=enum16{"Intialize", "Write", "Read", "Clear"}."Read") -> ("Cool-down time (s)"=w91:dbl, "Enable cool-down time"=w92:bool)  [unwired: 12 in, 1 out]
      n43 = Unbundle By Name(w99) -> ("Functional Mode"=w116:T16, "Number of POI"=w114:u16, "Number of Miniscans"=w113:u16, "Number of Cycles"=w112:u64, "Number of Trials"=w111:u16, "Miniscan Dwell time per pixel (us)"=w110:dbl, "Number of Pixels in Miniscan"=w109:u16, "POI Dwell time (us)"=w108:dbl, "Rectangle ROI length (pixels)"=w107:u16, "Rectangle ROI height (pixels)"=w106:u16, "AOL Mode"=w105:T17, "Plane Mode"=w104:T18, "Acquisition Length (sec)"=w103:dbl)
      n44 = global read "gl_Pockels control globals.vi" "Funct. acq. pockels modulation?"() -> (w115:bool)
      n45 = call "Experiment header-bundle basic image meta data.vi"("AOL_Globals"=w99) -> ("Basic image meta-data"=w119:T12)  [unwired: 10 in]
      n46 = call "fgv_total_roi_time.vi"("Op"=FGV_ROI_Time_Ops."Read") -> ("Cycle Rate"=w90:dbl)  [unwired: 6 in, 4 out]
      n47 = call "fgv_StimTrigFunct-Setup.vi"("Function"=enum16{"Intialize", "Write", "Read", "Clear"}."Read") -> ("Funct stim.trig.enable"=w95:bool, "Funct stim.trig.delay (sec)"=w96:dbl)  [unwired: 11 in, 2 out]
      n48 = Unbundle By Name(w99) -> ("Z Start"=w101:dbl, "Z Stop"=w100:dbl)
      n49 = Bundle By Name(cluster=T15 {"Functional Mode"=enum."Point", "Variable Length"=FALSE, "Variable Resolution"=FALSE, "Pockels Modulation"=FALSE, "Stimuli Trigger"=FALSE, "Cool down enabled"=FALSE, "AOL Mode"=enum."Raster", "Plane Mode"=0, "Miniscan Dwell time per pixel (us)"=0.0, "poi dwell time"=0.0, "Number of trials"=0.0, "Number of cycles"=0.0, "Number of pois"=0.0, "Number of miniscans"=0.0, "Number of pixels in miniscan"=0.0, "Rectangle ROI length"=0.0, "Rectangle ROI height"=0.0, "Frame rate (fps)"=0.0, "Acquisition Length"=0.0, "video length (sec)"=0.0, "Stimuli delay (sec)"=0.0, "Cool down time (sec)"=0.0, "Basic Image meta data"={"Wavelength (nm)"=0.0, "# averaged frames"=0.0, "laser power (%)"=0.0, "Pockels"=0.0, "pixel dwell time (us)"=0.0, "pmt 1"=0.0, "pmt 2"=0.0, "back apperture"=0.0, "zoom"=0.0, "field of view"=0.0, "Frame Size"=0, "AOL x centre"=0.0, "AOL y centre"=0.0, "Stage x position"=0.0, "Stage y position"=0.0, "Stage z position"=0.0}, "Z Start (um)"=0.0, "Z Stop (um)"=0.0} ("FUNCTIONAL IMAGING"), "Pockels Modulation"=w115, "Functional Mode"=w116, "Number of pois"=w114, "Number of miniscans"=w113, "Number of cycles"=w112, "Number of trials"=w111, "Miniscan Dwell time per pixel (us)"=w110, "Number of pixels in miniscan"=w109, "poi dwell time"=w108, "Rectangle ROI length"=w107, "Rectangle ROI height"=w106, "AOL Mode"=w105, "Plane Mode"=w104, "Acquisition Length"=w103, "Frame rate (fps)"=w90, "Stimuli Trigger"=w95, "Stimuli delay (sec)"=w96, "video length (sec)"=0.0, "Basic Image meta data"=w119, "Z Start (um)"=w101, "Z Stop (um)"=w100, "Variable Length"=w98, "Variable Resolution"=w94, "Cool down enabled"=w92, "Cool down time (sec)"=w91) -> (w117:T15)
      n50 = Bundle By Name(cluster=T6 {"LOGIN"={"User"="", "Profile"="", "Software Version"="", "Experiment Date Time"=timestamp(0 s since 1904-01-01)}, "GLOBAL PARAMETERS"={"MicroscopeID"="", "Microscope Type"="", "Objective"="", "Field of View (um)"=0.0, "Fill time (us)"=0.0, "Experiment Type"=enum."In vivo", "Stimuli Trigger"=FALSE, "Speed Logging"=FALSE}, "IMAGING MODES"={"Time Series"=FALSE, "Motor Zstack"=FALSE, "AOL Zstack"=FALSE, "Functional Imaging"=FALSE, "Volume Imaging"=FALSE}, "TIME SERIES"={"Basic Image meta data"={"Wavelength (nm)"=0.0, "# averaged frames"=0.0, "laser power (%)"=0.0, "Pockels"=0.0, "pixel dwell time (us)"=0.0, "pmt 1"=0.0, "pmt 2"=0.0, "back apperture"=0.0, "zoom"=0.0, "field of view"=0.0, "Frame Size"=0, "AOL x centre"=0.0, "AOL y centre"=0.0, "Stage x position"=0.0, "Stage y position"=0.0, "Stage z position"=0.0}, "AOL z"=0.0}, "MOTOR Z-STACK "={"Hdr Basic Image meta data"={"Wavelength (nm)"=0.0, "# averaged frames"=0.0, "laser power (%)"=0.0, "Pockels"=0.0, "pixel dwell time (us)"=0.0, "pmt 1"=0.0, "pmt 2"=0.0, "back apperture"=0.0, "zoom"=0.0, "field of view"=0.0, "Frame Size"=0, "AOL x centre"=0.0, "AOL y centre"=0.0, "Stage x position"=0.0, "Stage y position"=0.0, "Stage z position"=0.0}, "Z Start"=0.0, "Z Stop"=0.0, "No of Planes"=0, "Laser Power (%) at Z Start"=0.0, "Laser Power (%) at Z Stop"=0.0}, "AOL Z-STACK"={"Hdr Basic Image meta data"={"Wavelength (nm)"=0.0, "# averaged frames"=0.0, "laser power (%)"=0.0, "Pockels"=0.0, "pixel dwell time (us)"=0.0, "pmt 1"=0.0, "pmt 2"=0.0, "back apperture"=0.0, "zoom"=0.0, "field of view"=0.0, "Frame Size"=0, "AOL x centre"=0.0, "AOL y centre"=0.0, "Stage x position"=0.0, "Stage y position"=0.0, "Stage z position"=0.0}, "Z Start"=0.0, "Z Stop"=0.0, "No of Planes"=0, "Laser Power (%) at Z Start"=0.0, "Laser Power (%) at Z Stop"=0.0}, "FUNCTIONAL IMAGING"={"Functional Mode"=enum."Point", "Variable Length"=FALSE, "Variable Resolution"=FALSE, "Pockels Modulation"=FALSE, "Stimuli Trigger"=FALSE, "Cool down enabled"=FALSE, "AOL Mode"=enum."Raster", "Plane Mode"=0, "Miniscan Dwell time per pixel (us)"=0.0, "poi dwell time"=0.0, "Number of trials"=0.0, "Number of cycles"=0.0, "Number of pois"=0.0, "Number of miniscans"=0.0, "Number of pixels in miniscan"=0.0, "Rectangle ROI length"=0.0, "Rectangle ROI height"=0.0, "Frame rate (fps)"=0.0, "Acquisition Length"=0.0, "video length (sec)"=0.0, "Stimuli delay (sec)"=0.0, "Cool down time (sec)"=0.0, "Basic Image meta data"={"Wavelength (nm)"=0.0, "# averaged frames"=0.0, "laser power (%)"=0.0, "Pockels"=0.0, "pixel dwell time (us)"=0.0, "pmt 1"=0.0, "pmt 2"=0.0, "back apperture"=0.0, "zoom"=0.0, "field of view"=0.0, "Frame Size"=0, "AOL x centre"=0.0, "AOL y centre"=0.0, "Stage x position"=0.0, "Stage y position"=0.0, "Stage z position"=0.0}, "Z Start (um)"=0.0, "Z Stop (um)"=0.0}, "VOLUME IMAGING"={"Functional Mode"=enum."Point", "Variable Length"=FALSE, "Variable Resolution"=FALSE, "Pockels Modulation"=FALSE, "Stimuli Trigger"=FALSE, "Cool down enabled"=FALSE, "AOL Mode"=enum."Raster", "Plane Mode"=0, "Miniscan Dwell time per pixel (us)"=0.0, "poi dwell time"=0.0, "Number of trials"=0.0, "Number of cycles"=0.0, "Number of pois"=0.0, "Number of miniscans"=0.0, "Number of pixels in miniscan"=0.0, "Rectangle ROI length"=0.0, "Rectangle ROI height"=0.0, "Frame rate (fps)"=0.0, "Acquisition Length"=0.0, "video length (sec)"=0.0, "Stimuli delay (sec)"=0.0, "Cool down time (sec)"=0.0, "Basic Image meta data"={"Wavelength (nm)"=0.0, "# averaged frames"=0.0, "laser power (%)"=0.0, "Pockels"=0.0, "pixel dwell time (us)"=0.0, "pmt 1"=0.0, "pmt 2"=0.0, "back apperture"=0.0, "zoom"=0.0, "field of view"=0.0, "Frame Size"=0, "AOL x centre"=0.0, "AOL y centre"=0.0, "Stage x position"=0.0, "Stage y position"=0.0, "Stage z position"=0.0}, "Z Start (um)"=0.0, "Z Stop (um)"=0.0}, "MOVEMENT CORRECTION"={"Movement Correction"=FALSE, "Axial Reference"=FALSE, "Reference Source"=enum."Green channel", "Full Frame Size"=0.0, "Reference Field of View"=0.0, "Reference Zoom"=0.0, "Reference dwell time (us)"=0.0, "Reference X Pixels"=0.0, "Reference Y Pixels"=0.0, "Number of Z lines"=0.0, "Size of Z pixels"=0.0, "Axial Pixels"=0.0, "Ignore Z lines"=0.0, "Reference Scan Cycles"=0.0, "Reference Threshold XY"=0.0, "Reference Threshold Z"=0.0, "Reference Average XY"=0.0, "Reference Average Z"=0.0, "Proportional Scale"=0.0, "Integral Scale"=0.0, "Proportional Scale Z"=0.0, "Integral Scale Z"=0.0, "Diff Threshold"=0.0, "Diff Threshold Z"=0.0, "Sliding Average"=FALSE, "Reference count reset enabled"=FALSE, "Scan Interval (ms)"=0.0, "Ref Plot Refresh Rate (ms)"=0.0}, "CALIBRATION"={"Pockels Calibration File"=path "", "Calibration_ini file"=path "", "Setup_ini file"=path ""}, "STATISTICS"={"Z-stack duration (sec)"=0.0, "Number of acquired data-points"=0.0, "Acquisition time (ms)"=0.0, "Number of acquired frames"=0.0, "Intertrial times"=[]}, "BIOLOGY INFORMATION"={"Animal Code or Name"="", "Animal DoB"="", "Animal Age"="", "Animal Sex"="", "Animal Weight"="", "Date of Injection"="", "Date of Implant"="", "Site of Injection"="", "Animal Ear Notch"="", "AAV constructs"="", "Genetic background"="", "Optical reporter"="", "Region of brain imaged"="", "Other \ncomments"=""}, "Calibration Data"={"Objective Name"="", "Calibration Wavelength"=0.0, "Sum X"=0.0, "Sum Y"=0.0, "Diff X"=0.0, "Diff Y"=0.0, "Distortion Correction"=0.0, " Z norm to um Scaling"=0.0, " X norm to um Scaling"=0.0}} ("All header parameters in"), "FUNCTIONAL IMAGING"=w117) -> (w118:T6)
    }
    frame "VOLUME IMAGING" {
      n51 = Unbundle By Name(w130) -> ("Use Variable Length"=w129:bool, "Use Variable Resolution"=w122:bool)
      n52 = Unbundle By Name(w130) -> ("Functional Mode"=w150:T16, "Number of POI"=w148:u16, "Number of Miniscans"=w147:u16, "Number of Cycles"=w146:u64, "Number of Trials"=w145:u16, "Miniscan Dwell time per pixel (us)"=w144:dbl, "Number of Pixels in Miniscan"=w143:u16, "POI Dwell time (us)"=w142:dbl, "Rectangle ROI length (pixels)"=w141:u16, "Rectangle ROI height (pixels)"=w140:u16, "AOL Mode"=w139:T17, "Plane Mode"=w138:T18, "Acquisition Length (sec)"=w137:dbl)
      n53 = global read "gl_Pockels control globals.vi" "Funct. acq. pockels modulation?"() -> (w149:bool)
      n54 = call "Experiment header-Calculate frame rate.vi"("AOL_Globals"=w130) -> ("FrameRate (fps)"=w135:dbl)  [unwired: 10 in]
      n55 = call "fgv_StimTrigFunct-Setup.vi"("Function"=enum16{"Intialize", "Write", "Read", "Clear"}."Read") -> ("Funct stim.trig.enable"=w126:bool, "Funct stim.trig.width (ms)"=w127:dbl)  [unwired: 11 in, 2 out]
      n56 = call "Experiment header-bundle basic image meta data.vi"("AOL_Globals"=w130) -> ("Basic image meta-data"=w152:T12)  [unwired: 10 in]
      n57 = Unbundle By Name(w130) -> ("Z Start"=w134:dbl, "Z Stop"=w133:dbl)
      n58 = call "fgv_Cool down setup.vi"("Function"=enum16{"Intialize", "Write", "Read", "Clear"}."Read") -> ("Cool-down time (s)"=w123:dbl, "Enable cool-down time"=w124:bool)  [unwired: 12 in, 1 out]
      n59 = Bundle By Name(cluster=T15 {"Functional Mode"=enum."Point", "Variable Length"=FALSE, "Variable Resolution"=FALSE, "Pockels Modulation"=FALSE, "Stimuli Trigger"=FALSE, "Cool down enabled"=FALSE, "AOL Mode"=enum."Raster", "Plane Mode"=0, "Miniscan Dwell time per pixel (us)"=0.0, "poi dwell time"=0.0, "Number of trials"=0.0, "Number of cycles"=0.0, "Number of pois"=0.0, "Number of miniscans"=0.0, "Number of pixels in miniscan"=0.0, "Rectangle ROI length"=0.0, "Rectangle ROI height"=0.0, "Frame rate (fps)"=0.0, "Acquisition Length"=0.0, "video length (sec)"=0.0, "Stimuli delay (sec)"=0.0, "Cool down time (sec)"=0.0, "Basic Image meta data"={"Wavelength (nm)"=0.0, "# averaged frames"=0.0, "laser power (%)"=0.0, "Pockels"=0.0, "pixel dwell time (us)"=0.0, "pmt 1"=0.0, "pmt 2"=0.0, "back apperture"=0.0, "zoom"=0.0, "field of view"=0.0, "Frame Size"=0, "AOL x centre"=0.0, "AOL y centre"=0.0, "Stage x position"=0.0, "Stage y position"=0.0, "Stage z position"=0.0}, "Z Start (um)"=0.0, "Z Stop (um)"=0.0} ("FUNCTIONAL IMAGING"), "Pockels Modulation"=w149, "Functional Mode"=w150, "Number of pois"=w148, "Number of miniscans"=w147, "Number of cycles"=w146, "Number of trials"=w145, "Miniscan Dwell time per pixel (us)"=w144, "Number of pixels in miniscan"=w143, "poi dwell time"=w142, "Rectangle ROI length"=w141, "Rectangle ROI height"=w140, "AOL Mode"=w139, "Plane Mode"=w138, "Acquisition Length"=w137, "Frame rate (fps)"=w135, "Stimuli Trigger"=w126, "Stimuli delay (sec)"=w127, "video length (sec)"=0.0, "Basic Image meta data"=w152, "Z Start (um)"=w134, "Z Stop (um)"=w133, "Variable Length"=w129, "Variable Resolution"=w122, "Cool down enabled"=w124, "Cool down time (sec)"=w123) -> (w131:T15)
      n60 = Bundle By Name(cluster=T6 {"LOGIN"={"User"="", "Profile"="", "Software Version"="", "Experiment Date Time"=timestamp(0 s since 1904-01-01)}, "GLOBAL PARAMETERS"={"MicroscopeID"="", "Microscope Type"="", "Objective"="", "Field of View (um)"=0.0, "Fill time (us)"=0.0, "Experiment Type"=enum."In vivo", "Stimuli Trigger"=FALSE, "Speed Logging"=FALSE}, "IMAGING MODES"={"Time Series"=FALSE, "Motor Zstack"=FALSE, "AOL Zstack"=FALSE, "Functional Imaging"=FALSE, "Volume Imaging"=FALSE}, "TIME SERIES"={"Basic Image meta data"={"Wavelength (nm)"=0.0, "# averaged frames"=0.0, "laser power (%)"=0.0, "Pockels"=0.0, "pixel dwell time (us)"=0.0, "pmt 1"=0.0, "pmt 2"=0.0, "back apperture"=0.0, "zoom"=0.0, "field of view"=0.0, "Frame Size"=0, "AOL x centre"=0.0, "AOL y centre"=0.0, "Stage x position"=0.0, "Stage y position"=0.0, "Stage z position"=0.0}, "AOL z"=0.0}, "MOTOR Z-STACK "={"Hdr Basic Image meta data"={"Wavelength (nm)"=0.0, "# averaged frames"=0.0, "laser power (%)"=0.0, "Pockels"=0.0, "pixel dwell time (us)"=0.0, "pmt 1"=0.0, "pmt 2"=0.0, "back apperture"=0.0, "zoom"=0.0, "field of view"=0.0, "Frame Size"=0, "AOL x centre"=0.0, "AOL y centre"=0.0, "Stage x position"=0.0, "Stage y position"=0.0, "Stage z position"=0.0}, "Z Start"=0.0, "Z Stop"=0.0, "No of Planes"=0, "Laser Power (%) at Z Start"=0.0, "Laser Power (%) at Z Stop"=0.0}, "AOL Z-STACK"={"Hdr Basic Image meta data"={"Wavelength (nm)"=0.0, "# averaged frames"=0.0, "laser power (%)"=0.0, "Pockels"=0.0, "pixel dwell time (us)"=0.0, "pmt 1"=0.0, "pmt 2"=0.0, "back apperture"=0.0, "zoom"=0.0, "field of view"=0.0, "Frame Size"=0, "AOL x centre"=0.0, "AOL y centre"=0.0, "Stage x position"=0.0, "Stage y position"=0.0, "Stage z position"=0.0}, "Z Start"=0.0, "Z Stop"=0.0, "No of Planes"=0, "Laser Power (%) at Z Start"=0.0, "Laser Power (%) at Z Stop"=0.0}, "FUNCTIONAL IMAGING"={"Functional Mode"=enum."Point", "Variable Length"=FALSE, "Variable Resolution"=FALSE, "Pockels Modulation"=FALSE, "Stimuli Trigger"=FALSE, "Cool down enabled"=FALSE, "AOL Mode"=enum."Raster", "Plane Mode"=0, "Miniscan Dwell time per pixel (us)"=0.0, "poi dwell time"=0.0, "Number of trials"=0.0, "Number of cycles"=0.0, "Number of pois"=0.0, "Number of miniscans"=0.0, "Number of pixels in miniscan"=0.0, "Rectangle ROI length"=0.0, "Rectangle ROI height"=0.0, "Frame rate (fps)"=0.0, "Acquisition Length"=0.0, "video length (sec)"=0.0, "Stimuli delay (sec)"=0.0, "Cool down time (sec)"=0.0, "Basic Image meta data"={"Wavelength (nm)"=0.0, "# averaged frames"=0.0, "laser power (%)"=0.0, "Pockels"=0.0, "pixel dwell time (us)"=0.0, "pmt 1"=0.0, "pmt 2"=0.0, "back apperture"=0.0, "zoom"=0.0, "field of view"=0.0, "Frame Size"=0, "AOL x centre"=0.0, "AOL y centre"=0.0, "Stage x position"=0.0, "Stage y position"=0.0, "Stage z position"=0.0}, "Z Start (um)"=0.0, "Z Stop (um)"=0.0}, "VOLUME IMAGING"={"Functional Mode"=enum."Point", "Variable Length"=FALSE, "Variable Resolution"=FALSE, "Pockels Modulation"=FALSE, "Stimuli Trigger"=FALSE, "Cool down enabled"=FALSE, "AOL Mode"=enum."Raster", "Plane Mode"=0, "Miniscan Dwell time per pixel (us)"=0.0, "poi dwell time"=0.0, "Number of trials"=0.0, "Number of cycles"=0.0, "Number of pois"=0.0, "Number of miniscans"=0.0, "Number of pixels in miniscan"=0.0, "Rectangle ROI length"=0.0, "Rectangle ROI height"=0.0, "Frame rate (fps)"=0.0, "Acquisition Length"=0.0, "video length (sec)"=0.0, "Stimuli delay (sec)"=0.0, "Cool down time (sec)"=0.0, "Basic Image meta data"={"Wavelength (nm)"=0.0, "# averaged frames"=0.0, "laser power (%)"=0.0, "Pockels"=0.0, "pixel dwell time (us)"=0.0, "pmt 1"=0.0, "pmt 2"=0.0, "back apperture"=0.0, "zoom"=0.0, "field of view"=0.0, "Frame Size"=0, "AOL x centre"=0.0, "AOL y centre"=0.0, "Stage x position"=0.0, "Stage y position"=0.0, "Stage z position"=0.0}, "Z Start (um)"=0.0, "Z Stop (um)"=0.0}, "MOVEMENT CORRECTION"={"Movement Correction"=FALSE, "Axial Reference"=FALSE, "Reference Source"=enum."Green channel", "Full Frame Size"=0.0, "Reference Field of View"=0.0, "Reference Zoom"=0.0, "Reference dwell time (us)"=0.0, "Reference X Pixels"=0.0, "Reference Y Pixels"=0.0, "Number of Z lines"=0.0, "Size of Z pixels"=0.0, "Axial Pixels"=0.0, "Ignore Z lines"=0.0, "Reference Scan Cycles"=0.0, "Reference Threshold XY"=0.0, "Reference Threshold Z"=0.0, "Reference Average XY"=0.0, "Reference Average Z"=0.0, "Proportional Scale"=0.0, "Integral Scale"=0.0, "Proportional Scale Z"=0.0, "Integral Scale Z"=0.0, "Diff Threshold"=0.0, "Diff Threshold Z"=0.0, "Sliding Average"=FALSE, "Reference count reset enabled"=FALSE, "Scan Interval (ms)"=0.0, "Ref Plot Refresh Rate (ms)"=0.0}, "CALIBRATION"={"Pockels Calibration File"=path "", "Calibration_ini file"=path "", "Setup_ini file"=path ""}, "STATISTICS"={"Z-stack duration (sec)"=0.0, "Number of acquired data-points"=0.0, "Acquisition time (ms)"=0.0, "Number of acquired frames"=0.0, "Intertrial times"=[]}, "BIOLOGY INFORMATION"={"Animal Code or Name"="", "Animal DoB"="", "Animal Age"="", "Animal Sex"="", "Animal Weight"="", "Date of Injection"="", "Date of Implant"="", "Site of Injection"="", "Animal Ear Notch"="", "AAV constructs"="", "Genetic background"="", "Optical reporter"="", "Region of brain imaged"="", "Other \ncomments"=""}, "Calibration Data"={"Objective Name"="", "Calibration Wavelength"=0.0, "Sum X"=0.0, "Sum Y"=0.0, "Diff X"=0.0, "Diff Y"=0.0, "Distortion Correction"=0.0, " Z norm to um Scaling"=0.0, " X norm to um Scaling"=0.0}} ("All header parameters in"), "VOLUME IMAGING"=w131) -> (w151:T6)
      n61 = disable-structure shown="Disabled" {
        frame Disabled {
          (unwired) T29 {"Functional Mode"=enum."Point", "Pockels Modulation"=FALSE, "Number of pois"=0.0, "Number of miniscans"=0.0, "Number of cycles"=0.0, "Number of trials"=0.0, "Miniscan dwell time per pixel (us)"=0.0, "Number of pixels in miniscan"=0.0, "poi dwell time"=0.0, "Rectangle ROI length"=0.0, "Rectangle ROI height"=0.0, "AOL Mode"=enum."Raster", "Plane Mode"=0, "video length (sec)"=0.0, "Frame rate (fps)"=0.0, "Stimuli Timing (usec)"=0.0, "Acquisition Length"=0.0, "Basic Image meta data"={"Wavelength (nm)"=0.0, "# averaged frames"=0.0, "laser power (%)"=0.0, "Pockels"=0.0, "pixel dwell time (us)"=0.0, "pmt 1"=0.0, "pmt 2"=0.0, "back apperture"=0.0, "zoom"=0.0, "field of view"=0.0, "Frame Size"=0, "AOL x centre"=0.0, "AOL y centre"=0.0, "Stage x position"=0.0, "Stage y position"=0.0, "Stage z position"=0.0}, "Z Start (um)"=0.0, "Z Stop (um)"=0.0} ("FUNCTIONAL IMAGING")
        }
        frame Enabled {
        }
      }
    }
    frame "MOVEMENT CORRECTION" {
      n62 = call "fgv_RefDAQParam.vi"("Function"=enum16{"Initialize", "Write", "Read"}."Read") -> ("RefDAQParam"=w195:T30)  [unwired: 9 in, 1 out]
      n63 = global read "gl_UI Ctrl Refs.vi" "UI ctrl refs"() -> (w194:T27)
      n64 = Unbundle By Name(w195) -> ("Full Frame Size"=w156:u16, "Ref Field of View"=w155:sgl, "Ref Zoom"=w154:i8, "Ref_dwellTime"=w186:sgl, "Ref X-pixels-per-line(Npxr)"=w185:i16, "Ref Y-lines-per-image(Npyr)"=w184:i16, "Ref Z-lines-per-image"=w183:i16, "Ignore Z lines"=w179:i16, "Ref Scan Cycles"=w178:i32, "Ref threshold XY"=w177:u16, "Ref threshold Z"=w176:u16, "Ref average XY"=w175:u16, "Ref Average  Z"=w174:u16, "Proportional_scale"=w171:fxp<+,16,2>, "Integral_scale"=w169:fxp<+/-,16,12>, "Proportional_scale Z"=w167:fxp<+,16,2>, "Integral_scale Z"=w165:fxp<+/-,16,12>, "Diff_threshold"=w163:fxp<+,16,2>, "Diff_threshold _z"=w162:fxp<+,16,2>, "Sliding Average"=w173:bool, "Ref count reset enabled"=w172:bool)
      n65 = Unbundle By Name(w194) -> ("Reference Source"=w193:refnum<vi>)
      n66 = global read "gl_Pockels control globals.vi" "Target time between mov.cor. ref triggers (ms)"() -> (w159:dbl)
      n67 = global read "General Globals.vi" "Movement Correction"() -> (w190:bool)
      n68 = property class="Enum (strict)"(reference=w193) -> ("Value"=w187:enum16{"Green channel", "Red channel"})  [unwired: 1 in, 2 out]
      n69 = global read "General Globals.vi" "Axial Scanning"() -> (w188:bool)
      n70 = global read "gl_RefPlotRefreshRate.vi" "Ref Plot refresh rate"() -> (w158:dbl)
      n71 = To Double Precision Float(number=w163) -> (double precision float=w161:dbl)
      n72 = To Double Precision Float(number=w162) -> (double precision float=w160:dbl)
      n73 = To Double Precision Float(number=w171) -> (double precision float=w170:dbl)
      n74 = To Double Precision Float(number=w169) -> (double precision float=w168:dbl)
      n75 = To Double Precision Float(number=w167) -> (double precision float=w166:dbl)
      n76 = To Double Precision Float(number=w165) -> (double precision float=w164:dbl)
      n77 = call "fgv_Reference_Globals.vi"("Function"=enum16{"Intialize", "Write", "Read", "Clear"}."Read") -> ("Reference Data"=w182:T31)  [unwired: 9 in, 1 out]
      n78 = Unbundle By Name(w182) -> ("Z Step"=w181:i8, "Z pixels"=w180:i32)
      n79 = Bundle By Name(cluster=T19 {"Movement Correction"=FALSE, "Axial Reference"=FALSE, "Reference Source"=enum."Green channel", "Full Frame Size"=0.0, "Reference Field of View"=0.0, "Reference Zoom"=0.0, "Reference dwell time (us)"=0.0, "Reference X Pixels"=0.0, "Reference Y Pixels"=0.0, "Number of Z lines"=0.0, "Size of Z pixels"=0.0, "Axial Pixels"=0.0, "Ignore Z lines"=0.0, "Reference Scan Cycles"=0.0, "Reference Threshold XY"=0.0, "Reference Threshold Z"=0.0, "Reference Average XY"=0.0, "Reference Average Z"=0.0, "Proportional Scale"=0.0, "Integral Scale"=0.0, "Proportional Scale Z"=0.0, "Integral Scale Z"=0.0, "Diff Threshold"=0.0, "Diff Threshold Z"=0.0, "Sliding Average"=FALSE, "Reference count reset enabled"=FALSE, "Scan Interval (ms)"=0.0, "Ref Plot Refresh Rate (ms)"=0.0} ("MOVEMENT CORRECTION"), "Movement Correction"=w190, "Axial Reference"=w188, "Reference Source"=w187, "Full Frame Size"=w156, "Reference Field of View"=w155, "Reference Zoom"=w154, "Reference dwell time (us)"=w186, "Reference X Pixels"=w185, "Reference Y Pixels"=w184, "Number of Z lines"=w183, "Size of Z pixels"=w181, "Axial Pixels"=w180, "Ignore Z lines"=w179, "Reference Scan Cycles"=w178, "Reference Threshold XY"=w177, "Reference Threshold Z"=w176, "Reference Average XY"=w175, "Reference Average Z"=w174, "Proportional Scale"=w170, "Integral Scale"=w168, "Proportional Scale Z"=w166, "Integral Scale Z"=w164, "Diff Threshold"=w161, "Diff Threshold Z"=w160, "Sliding Average"=w173, "Reference count reset enabled"=w172, "Scan Interval (ms)"=w159, "Ref Plot Refresh Rate (ms)"=w158) -> (w189:T19)
      n80 = Bundle By Name(cluster=T6 {"LOGIN"={"User"="", "Profile"="", "Software Version"="", "Experiment Date Time"=timestamp(0 s since 1904-01-01)}, "GLOBAL PARAMETERS"={"MicroscopeID"="", "Microscope Type"="", "Objective"="", "Field of View (um)"=0.0, "Fill time (us)"=0.0, "Experiment Type"=enum."In vivo", "Stimuli Trigger"=FALSE, "Speed Logging"=FALSE}, "IMAGING MODES"={"Time Series"=FALSE, "Motor Zstack"=FALSE, "AOL Zstack"=FALSE, "Functional Imaging"=FALSE, "Volume Imaging"=FALSE}, "TIME SERIES"={"Basic Image meta data"={"Wavelength (nm)"=0.0, "# averaged frames"=0.0, "laser power (%)"=0.0, "Pockels"=0.0, "pixel dwell time (us)"=0.0, "pmt 1"=0.0, "pmt 2"=0.0, "back apperture"=0.0, "zoom"=0.0, "field of view"=0.0, "Frame Size"=0, "AOL x centre"=0.0, "AOL y centre"=0.0, "Stage x position"=0.0, "Stage y position"=0.0, "Stage z position"=0.0}, "AOL z"=0.0}, "MOTOR Z-STACK "={"Hdr Basic Image meta data"={"Wavelength (nm)"=0.0, "# averaged frames"=0.0, "laser power (%)"=0.0, "Pockels"=0.0, "pixel dwell time (us)"=0.0, "pmt 1"=0.0, "pmt 2"=0.0, "back apperture"=0.0, "zoom"=0.0, "field of view"=0.0, "Frame Size"=0, "AOL x centre"=0.0, "AOL y centre"=0.0, "Stage x position"=0.0, "Stage y position"=0.0, "Stage z position"=0.0}, "Z Start"=0.0, "Z Stop"=0.0, "No of Planes"=0, "Laser Power (%) at Z Start"=0.0, "Laser Power (%) at Z Stop"=0.0}, "AOL Z-STACK"={"Hdr Basic Image meta data"={"Wavelength (nm)"=0.0, "# averaged frames"=0.0, "laser power (%)"=0.0, "Pockels"=0.0, "pixel dwell time (us)"=0.0, "pmt 1"=0.0, "pmt 2"=0.0, "back apperture"=0.0, "zoom"=0.0, "field of view"=0.0, "Frame Size"=0, "AOL x centre"=0.0, "AOL y centre"=0.0, "Stage x position"=0.0, "Stage y position"=0.0, "Stage z position"=0.0}, "Z Start"=0.0, "Z Stop"=0.0, "No of Planes"=0, "Laser Power (%) at Z Start"=0.0, "Laser Power (%) at Z Stop"=0.0}, "FUNCTIONAL IMAGING"={"Functional Mode"=enum."Point", "Variable Length"=FALSE, "Variable Resolution"=FALSE, "Pockels Modulation"=FALSE, "Stimuli Trigger"=FALSE, "Cool down enabled"=FALSE, "AOL Mode"=enum."Raster", "Plane Mode"=0, "Miniscan Dwell time per pixel (us)"=0.0, "poi dwell time"=0.0, "Number of trials"=0.0, "Number of cycles"=0.0, "Number of pois"=0.0, "Number of miniscans"=0.0, "Number of pixels in miniscan"=0.0, "Rectangle ROI length"=0.0, "Rectangle ROI height"=0.0, "Frame rate (fps)"=0.0, "Acquisition Length"=0.0, "video length (sec)"=0.0, "Stimuli delay (sec)"=0.0, "Cool down time (sec)"=0.0, "Basic Image meta data"={"Wavelength (nm)"=0.0, "# averaged frames"=0.0, "laser power (%)"=0.0, "Pockels"=0.0, "pixel dwell time (us)"=0.0, "pmt 1"=0.0, "pmt 2"=0.0, "back apperture"=0.0, "zoom"=0.0, "field of view"=0.0, "Frame Size"=0, "AOL x centre"=0.0, "AOL y centre"=0.0, "Stage x position"=0.0, "Stage y position"=0.0, "Stage z position"=0.0}, "Z Start (um)"=0.0, "Z Stop (um)"=0.0}, "VOLUME IMAGING"={"Functional Mode"=enum."Point", "Variable Length"=FALSE, "Variable Resolution"=FALSE, "Pockels Modulation"=FALSE, "Stimuli Trigger"=FALSE, "Cool down enabled"=FALSE, "AOL Mode"=enum."Raster", "Plane Mode"=0, "Miniscan Dwell time per pixel (us)"=0.0, "poi dwell time"=0.0, "Number of trials"=0.0, "Number of cycles"=0.0, "Number of pois"=0.0, "Number of miniscans"=0.0, "Number of pixels in miniscan"=0.0, "Rectangle ROI length"=0.0, "Rectangle ROI height"=0.0, "Frame rate (fps)"=0.0, "Acquisition Length"=0.0, "video length (sec)"=0.0, "Stimuli delay (sec)"=0.0, "Cool down time (sec)"=0.0, "Basic Image meta data"={"Wavelength (nm)"=0.0, "# averaged frames"=0.0, "laser power (%)"=0.0, "Pockels"=0.0, "pixel dwell time (us)"=0.0, "pmt 1"=0.0, "pmt 2"=0.0, "back apperture"=0.0, "zoom"=0.0, "field of view"=0.0, "Frame Size"=0, "AOL x centre"=0.0, "AOL y centre"=0.0, "Stage x position"=0.0, "Stage y position"=0.0, "Stage z position"=0.0}, "Z Start (um)"=0.0, "Z Stop (um)"=0.0}, "MOVEMENT CORRECTION"={"Movement Correction"=FALSE, "Axial Reference"=FALSE, "Reference Source"=enum."Green channel", "Full Frame Size"=0.0, "Reference Field of View"=0.0, "Reference Zoom"=0.0, "Reference dwell time (us)"=0.0, "Reference X Pixels"=0.0, "Reference Y Pixels"=0.0, "Number of Z lines"=0.0, "Size of Z pixels"=0.0, "Axial Pixels"=0.0, "Ignore Z lines"=0.0, "Reference Scan Cycles"=0.0, "Reference Threshold XY"=0.0, "Reference Threshold Z"=0.0, "Reference Average XY"=0.0, "Reference Average Z"=0.0, "Proportional Scale"=0.0, "Integral Scale"=0.0, "Proportional Scale Z"=0.0, "Integral Scale Z"=0.0, "Diff Threshold"=0.0, "Diff Threshold Z"=0.0, "Sliding Average"=FALSE, "Reference count reset enabled"=FALSE, "Scan Interval (ms)"=0.0, "Ref Plot Refresh Rate (ms)"=0.0}, "CALIBRATION"={"Pockels Calibration File"=path "", "Calibration_ini file"=path "", "Setup_ini file"=path ""}, "STATISTICS"={"Z-stack duration (sec)"=0.0, "Number of acquired data-points"=0.0, "Acquisition time (ms)"=0.0, "Number of acquired frames"=0.0, "Intertrial times"=[]}, "BIOLOGY INFORMATION"={"Animal Code or Name"="", "Animal DoB"="", "Animal Age"="", "Animal Sex"="", "Animal Weight"="", "Date of Injection"="", "Date of Implant"="", "Site of Injection"="", "Animal Ear Notch"="", "AAV constructs"="", "Genetic background"="", "Optical reporter"="", "Region of brain imaged"="", "Other \ncomments"=""}, "Calibration Data"={"Objective Name"="", "Calibration Wavelength"=0.0, "Sum X"=0.0, "Sum Y"=0.0, "Diff X"=0.0, "Diff Y"=0.0, "Distortion Correction"=0.0, " Z norm to um Scaling"=0.0, " X norm to um Scaling"=0.0}} ("All header parameters in"), "MOVEMENT CORRECTION"=w189) -> (w192:T6)
    }
    frame "CALIBRATION" {
      n81 = global read "gl_Calibration globals.vi" "Pockels cal file name"() -> (w204:string)
      n82 = global read "General Globals.vi" "Config Files Folder Path"() -> (w202:path)
      n83 = Concatenate Strings("Calibration Files\\", w204) -> (w203:string)
      n84 = Build Path(base path=w202, name or relative path=w203) -> (appended path=w200:path)
      n85 = Build Path(base path=w202, name or relative path="Calibration.ini") -> (appended path=w201:path)
      n86 = Build Path(base path=w202, name or relative path="Setup.ini") -> (appended path=w207:path)
      n87 = Bundle By Name(cluster=T21 {"Pockels Calibration File"=path "", "Calibration_ini file"=path "", "Setup_ini file"=path ""} ("CALIBRATION"), "Pockels Calibration File"=w200, "Calibration_ini file"=w201, "Setup_ini file"=w207) -> (w199:T21)
      n88 = Bundle By Name(cluster=T6 {"LOGIN"={"User"="", "Profile"="", "Software Version"="", "Experiment Date Time"=timestamp(0 s since 1904-01-01)}, "GLOBAL PARAMETERS"={"MicroscopeID"="", "Microscope Type"="", "Objective"="", "Field of View (um)"=0.0, "Fill time (us)"=0.0, "Experiment Type"=enum."In vivo", "Stimuli Trigger"=FALSE, "Speed Logging"=FALSE}, "IMAGING MODES"={"Time Series"=FALSE, "Motor Zstack"=FALSE, "AOL Zstack"=FALSE, "Functional Imaging"=FALSE, "Volume Imaging"=FALSE}, "TIME SERIES"={"Basic Image meta data"={"Wavelength (nm)"=0.0, "# averaged frames"=0.0, "laser power (%)"=0.0, "Pockels"=0.0, "pixel dwell time (us)"=0.0, "pmt 1"=0.0, "pmt 2"=0.0, "back apperture"=0.0, "zoom"=0.0, "field of view"=0.0, "Frame Size"=0, "AOL x centre"=0.0, "AOL y centre"=0.0, "Stage x position"=0.0, "Stage y position"=0.0, "Stage z position"=0.0}, "AOL z"=0.0}, "MOTOR Z-STACK "={"Hdr Basic Image meta data"={"Wavelength (nm)"=0.0, "# averaged frames"=0.0, "laser power (%)"=0.0, "Pockels"=0.0, "pixel dwell time (us)"=0.0, "pmt 1"=0.0, "pmt 2"=0.0, "back apperture"=0.0, "zoom"=0.0, "field of view"=0.0, "Frame Size"=0, "AOL x centre"=0.0, "AOL y centre"=0.0, "Stage x position"=0.0, "Stage y position"=0.0, "Stage z position"=0.0}, "Z Start"=0.0, "Z Stop"=0.0, "No of Planes"=0, "Laser Power (%) at Z Start"=0.0, "Laser Power (%) at Z Stop"=0.0}, "AOL Z-STACK"={"Hdr Basic Image meta data"={"Wavelength (nm)"=0.0, "# averaged frames"=0.0, "laser power (%)"=0.0, "Pockels"=0.0, "pixel dwell time (us)"=0.0, "pmt 1"=0.0, "pmt 2"=0.0, "back apperture"=0.0, "zoom"=0.0, "field of view"=0.0, "Frame Size"=0, "AOL x centre"=0.0, "AOL y centre"=0.0, "Stage x position"=0.0, "Stage y position"=0.0, "Stage z position"=0.0}, "Z Start"=0.0, "Z Stop"=0.0, "No of Planes"=0, "Laser Power (%) at Z Start"=0.0, "Laser Power (%) at Z Stop"=0.0}, "FUNCTIONAL IMAGING"={"Functional Mode"=enum."Point", "Variable Length"=FALSE, "Variable Resolution"=FALSE, "Pockels Modulation"=FALSE, "Stimuli Trigger"=FALSE, "Cool down enabled"=FALSE, "AOL Mode"=enum."Raster", "Plane Mode"=0, "Miniscan Dwell time per pixel (us)"=0.0, "poi dwell time"=0.0, "Number of trials"=0.0, "Number of cycles"=0.0, "Number of pois"=0.0, "Number of miniscans"=0.0, "Number of pixels in miniscan"=0.0, "Rectangle ROI length"=0.0, "Rectangle ROI height"=0.0, "Frame rate (fps)"=0.0, "Acquisition Length"=0.0, "video length (sec)"=0.0, "Stimuli delay (sec)"=0.0, "Cool down time (sec)"=0.0, "Basic Image meta data"={"Wavelength (nm)"=0.0, "# averaged frames"=0.0, "laser power (%)"=0.0, "Pockels"=0.0, "pixel dwell time (us)"=0.0, "pmt 1"=0.0, "pmt 2"=0.0, "back apperture"=0.0, "zoom"=0.0, "field of view"=0.0, "Frame Size"=0, "AOL x centre"=0.0, "AOL y centre"=0.0, "Stage x position"=0.0, "Stage y position"=0.0, "Stage z position"=0.0}, "Z Start (um)"=0.0, "Z Stop (um)"=0.0}, "VOLUME IMAGING"={"Functional Mode"=enum."Point", "Variable Length"=FALSE, "Variable Resolution"=FALSE, "Pockels Modulation"=FALSE, "Stimuli Trigger"=FALSE, "Cool down enabled"=FALSE, "AOL Mode"=enum."Raster", "Plane Mode"=0, "Miniscan Dwell time per pixel (us)"=0.0, "poi dwell time"=0.0, "Number of trials"=0.0, "Number of cycles"=0.0, "Number of pois"=0.0, "Number of miniscans"=0.0, "Number of pixels in miniscan"=0.0, "Rectangle ROI length"=0.0, "Rectangle ROI height"=0.0, "Frame rate (fps)"=0.0, "Acquisition Length"=0.0, "video length (sec)"=0.0, "Stimuli delay (sec)"=0.0, "Cool down time (sec)"=0.0, "Basic Image meta data"={"Wavelength (nm)"=0.0, "# averaged frames"=0.0, "laser power (%)"=0.0, "Pockels"=0.0, "pixel dwell time (us)"=0.0, "pmt 1"=0.0, "pmt 2"=0.0, "back apperture"=0.0, "zoom"=0.0, "field of view"=0.0, "Frame Size"=0, "AOL x centre"=0.0, "AOL y centre"=0.0, "Stage x position"=0.0, "Stage y position"=0.0, "Stage z position"=0.0}, "Z Start (um)"=0.0, "Z Stop (um)"=0.0}, "MOVEMENT CORRECTION"={"Movement Correction"=FALSE, "Axial Reference"=FALSE, "Reference Source"=enum."Green channel", "Full Frame Size"=0.0, "Reference Field of View"=0.0, "Reference Zoom"=0.0, "Reference dwell time (us)"=0.0, "Reference X Pixels"=0.0, "Reference Y Pixels"=0.0, "Number of Z lines"=0.0, "Size of Z pixels"=0.0, "Axial Pixels"=0.0, "Ignore Z lines"=0.0, "Reference Scan Cycles"=0.0, "Reference Threshold XY"=0.0, "Reference Threshold Z"=0.0, "Reference Average XY"=0.0, "Reference Average Z"=0.0, "Proportional Scale"=0.0, "Integral Scale"=0.0, "Proportional Scale Z"=0.0, "Integral Scale Z"=0.0, "Diff Threshold"=0.0, "Diff Threshold Z"=0.0, "Sliding Average"=FALSE, "Reference count reset enabled"=FALSE, "Scan Interval (ms)"=0.0, "Ref Plot Refresh Rate (ms)"=0.0}, "CALIBRATION"={"Pockels Calibration File"=path "", "Calibration_ini file"=path "", "Setup_ini file"=path ""}, "STATISTICS"={"Z-stack duration (sec)"=0.0, "Number of acquired data-points"=0.0, "Acquisition time (ms)"=0.0, "Number of acquired frames"=0.0, "Intertrial times"=[]}, "BIOLOGY INFORMATION"={"Animal Code or Name"="", "Animal DoB"="", "Animal Age"="", "Animal Sex"="", "Animal Weight"="", "Date of Injection"="", "Date of Implant"="", "Site of Injection"="", "Animal Ear Notch"="", "AAV constructs"="", "Genetic background"="", "Optical reporter"="", "Region of brain imaged"="", "Other \ncomments"=""}, "Calibration Data"={"Objective Name"="", "Calibration Wavelength"=0.0, "Sum X"=0.0, "Sum Y"=0.0, "Diff X"=0.0, "Diff Y"=0.0, "Distortion Correction"=0.0, " Z norm to um Scaling"=0.0, " X norm to um Scaling"=0.0}} ("All header parameters in"), "CALIBRATION"=w199) -> (w198:T6)
    }
    frame "STATISTICS" {
      # "THE VALUES ARE CORRECT ONLY WHEN CALLED AFTER THE LAST\nTRIAL OR WHEN FUNCTIONAL IMAGING IS ABORTED.\nTHIS CASE SHOULD ONLY BE CALLED THEN"
      n89 = global read "General Globals.vi" "Timelapse frames saved"() -> (w220:u32)
      n90 = global read "General Globals.vi" "Protocol start timestamp"() -> (w213:timestamp)
      n91 = Get Date/Time In Seconds() -> (seconds since 1Jan1904=w214:timestamp)
      n92 = call "Experiment header-Calculate STATS.vi"("Logging queue element"=w219, "Timelapse frames saved"=w220) -> ("Number of acquired frames"=w215:dbl, "Acquisition time (ms)"=w216:dbl, "Total number of points acquired (Ch0)"=w217:dbl)  [unwired: 7 in]
      n93 = Subtract(x=w214, y=w213) -> (x-y=w212:dbl)
      n94 = Bundle By Name(cluster=T22 {"Z-stack duration (sec)"=0.0, "Number of acquired data-points"=0.0, "Acquisition time (ms)"=0.0, "Number of acquired frames"=0.0, "Intertrial times"=[]} ("STATISTICS"), "Z-stack duration (sec)"=w212, "Number of acquired data-points"=w217, "Acquisition time (ms)"=w216, "Number of acquired frames"=w215) -> (w211:T22)
      n95 = Bundle By Name(cluster=T6 {"LOGIN"={"User"="", "Profile"="", "Software Version"="", "Experiment Date Time"=timestamp(0 s since 1904-01-01)}, "GLOBAL PARAMETERS"={"MicroscopeID"="", "Microscope Type"="", "Objective"="", "Field of View (um)"=0.0, "Fill time (us)"=0.0, "Experiment Type"=enum."In vivo", "Stimuli Trigger"=FALSE, "Speed Logging"=FALSE}, "IMAGING MODES"={"Time Series"=FALSE, "Motor Zstack"=FALSE, "AOL Zstack"=FALSE, "Functional Imaging"=FALSE, "Volume Imaging"=FALSE}, "TIME SERIES"={"Basic Image meta data"={"Wavelength (nm)"=0.0, "# averaged frames"=0.0, "laser power (%)"=0.0, "Pockels"=0.0, "pixel dwell time (us)"=0.0, "pmt 1"=0.0, "pmt 2"=0.0, "back apperture"=0.0, "zoom"=0.0, "field of view"=0.0, "Frame Size"=0, "AOL x centre"=0.0, "AOL y centre"=0.0, "Stage x position"=0.0, "Stage y position"=0.0, "Stage z position"=0.0}, "AOL z"=0.0}, "MOTOR Z-STACK "={"Hdr Basic Image meta data"={"Wavelength (nm)"=0.0, "# averaged frames"=0.0, "laser power (%)"=0.0, "Pockels"=0.0, "pixel dwell time (us)"=0.0, "pmt 1"=0.0, "pmt 2"=0.0, "back apperture"=0.0, "zoom"=0.0, "field of view"=0.0, "Frame Size"=0, "AOL x centre"=0.0, "AOL y centre"=0.0, "Stage x position"=0.0, "Stage y position"=0.0, "Stage z position"=0.0}, "Z Start"=0.0, "Z Stop"=0.0, "No of Planes"=0, "Laser Power (%) at Z Start"=0.0, "Laser Power (%) at Z Stop"=0.0}, "AOL Z-STACK"={"Hdr Basic Image meta data"={"Wavelength (nm)"=0.0, "# averaged frames"=0.0, "laser power (%)"=0.0, "Pockels"=0.0, "pixel dwell time (us)"=0.0, "pmt 1"=0.0, "pmt 2"=0.0, "back apperture"=0.0, "zoom"=0.0, "field of view"=0.0, "Frame Size"=0, "AOL x centre"=0.0, "AOL y centre"=0.0, "Stage x position"=0.0, "Stage y position"=0.0, "Stage z position"=0.0}, "Z Start"=0.0, "Z Stop"=0.0, "No of Planes"=0, "Laser Power (%) at Z Start"=0.0, "Laser Power (%) at Z Stop"=0.0}, "FUNCTIONAL IMAGING"={"Functional Mode"=enum."Point", "Variable Length"=FALSE, "Variable Resolution"=FALSE, "Pockels Modulation"=FALSE, "Stimuli Trigger"=FALSE, "Cool down enabled"=FALSE, "AOL Mode"=enum."Raster", "Plane Mode"=0, "Miniscan Dwell time per pixel (us)"=0.0, "poi dwell time"=0.0, "Number of trials"=0.0, "Number of cycles"=0.0, "Number of pois"=0.0, "Number of miniscans"=0.0, "Number of pixels in miniscan"=0.0, "Rectangle ROI length"=0.0, "Rectangle ROI height"=0.0, "Frame rate (fps)"=0.0, "Acquisition Length"=0.0, "video length (sec)"=0.0, "Stimuli delay (sec)"=0.0, "Cool down time (sec)"=0.0, "Basic Image meta data"={"Wavelength (nm)"=0.0, "# averaged frames"=0.0, "laser power (%)"=0.0, "Pockels"=0.0, "pixel dwell time (us)"=0.0, "pmt 1"=0.0, "pmt 2"=0.0, "back apperture"=0.0, "zoom"=0.0, "field of view"=0.0, "Frame Size"=0, "AOL x centre"=0.0, "AOL y centre"=0.0, "Stage x position"=0.0, "Stage y position"=0.0, "Stage z position"=0.0}, "Z Start (um)"=0.0, "Z Stop (um)"=0.0}, "VOLUME IMAGING"={"Functional Mode"=enum."Point", "Variable Length"=FALSE, "Variable Resolution"=FALSE, "Pockels Modulation"=FALSE, "Stimuli Trigger"=FALSE, "Cool down enabled"=FALSE, "AOL Mode"=enum."Raster", "Plane Mode"=0, "Miniscan Dwell time per pixel (us)"=0.0, "poi dwell time"=0.0, "Number of trials"=0.0, "Number of cycles"=0.0, "Number of pois"=0.0, "Number of miniscans"=0.0, "Number of pixels in miniscan"=0.0, "Rectangle ROI length"=0.0, "Rectangle ROI height"=0.0, "Frame rate (fps)"=0.0, "Acquisition Length"=0.0, "video length (sec)"=0.0, "Stimuli delay (sec)"=0.0, "Cool down time (sec)"=0.0, "Basic Image meta data"={"Wavelength (nm)"=0.0, "# averaged frames"=0.0, "laser power (%)"=0.0, "Pockels"=0.0, "pixel dwell time (us)"=0.0, "pmt 1"=0.0, "pmt 2"=0.0, "back apperture"=0.0, "zoom"=0.0, "field of view"=0.0, "Frame Size"=0, "AOL x centre"=0.0, "AOL y centre"=0.0, "Stage x position"=0.0, "Stage y position"=0.0, "Stage z position"=0.0}, "Z Start (um)"=0.0, "Z Stop (um)"=0.0}, "MOVEMENT CORRECTION"={"Movement Correction"=FALSE, "Axial Reference"=FALSE, "Reference Source"=enum."Green channel", "Full Frame Size"=0.0, "Reference Field of View"=0.0, "Reference Zoom"=0.0, "Reference dwell time (us)"=0.0, "Reference X Pixels"=0.0, "Reference Y Pixels"=0.0, "Number of Z lines"=0.0, "Size of Z pixels"=0.0, "Axial Pixels"=0.0, "Ignore Z lines"=0.0, "Reference Scan Cycles"=0.0, "Reference Threshold XY"=0.0, "Reference Threshold Z"=0.0, "Reference Average XY"=0.0, "Reference Average Z"=0.0, "Proportional Scale"=0.0, "Integral Scale"=0.0, "Proportional Scale Z"=0.0, "Integral Scale Z"=0.0, "Diff Threshold"=0.0, "Diff Threshold Z"=0.0, "Sliding Average"=FALSE, "Reference count reset enabled"=FALSE, "Scan Interval (ms)"=0.0, "Ref Plot Refresh Rate (ms)"=0.0}, "CALIBRATION"={"Pockels Calibration File"=path "", "Calibration_ini file"=path "", "Setup_ini file"=path ""}, "STATISTICS"={"Z-stack duration (sec)"=0.0, "Number of acquired data-points"=0.0, "Acquisition time (ms)"=0.0, "Number of acquired frames"=0.0, "Intertrial times"=[]}, "BIOLOGY INFORMATION"={"Animal Code or Name"="", "Animal DoB"="", "Animal Age"="", "Animal Sex"="", "Animal Weight"="", "Date of Injection"="", "Date of Implant"="", "Site of Injection"="", "Animal Ear Notch"="", "AAV constructs"="", "Genetic background"="", "Optical reporter"="", "Region of brain imaged"="", "Other \ncomments"=""}, "Calibration Data"={"Objective Name"="", "Calibration Wavelength"=0.0, "Sum X"=0.0, "Sum Y"=0.0, "Diff X"=0.0, "Diff Y"=0.0, "Distortion Correction"=0.0, " Z norm to um Scaling"=0.0, " X norm to um Scaling"=0.0}} ("All header parameters in"), "STATISTICS"=w211) -> (w221:T6)
    }
    frame "BIOLOGY INFORMATION" {
      n96 = global read "gl_UI Ctrl Refs.vi" "UI ctrl refs"() -> (w226:T27)
      n97 = Unbundle By Name(w226) -> ("Biology Information"=w225:refnum<vi>)
      n98 = property class="Clust (strict)"(reference=w225) -> ("Value"=w224:T23)  [unwired: 1 in, 2 out]
      n99 = Bundle By Name(cluster=T6 {"LOGIN"={"User"="", "Profile"="", "Software Version"="", "Experiment Date Time"=timestamp(0 s since 1904-01-01)}, "GLOBAL PARAMETERS"={"MicroscopeID"="", "Microscope Type"="", "Objective"="", "Field of View (um)"=0.0, "Fill time (us)"=0.0, "Experiment Type"=enum."In vivo", "Stimuli Trigger"=FALSE, "Speed Logging"=FALSE}, "IMAGING MODES"={"Time Series"=FALSE, "Motor Zstack"=FALSE, "AOL Zstack"=FALSE, "Functional Imaging"=FALSE, "Volume Imaging"=FALSE}, "TIME SERIES"={"Basic Image meta data"={"Wavelength (nm)"=0.0, "# averaged frames"=0.0, "laser power (%)"=0.0, "Pockels"=0.0, "pixel dwell time (us)"=0.0, "pmt 1"=0.0, "pmt 2"=0.0, "back apperture"=0.0, "zoom"=0.0, "field of view"=0.0, "Frame Size"=0, "AOL x centre"=0.0, "AOL y centre"=0.0, "Stage x position"=0.0, "Stage y position"=0.0, "Stage z position"=0.0}, "AOL z"=0.0}, "MOTOR Z-STACK "={"Hdr Basic Image meta data"={"Wavelength (nm)"=0.0, "# averaged frames"=0.0, "laser power (%)"=0.0, "Pockels"=0.0, "pixel dwell time (us)"=0.0, "pmt 1"=0.0, "pmt 2"=0.0, "back apperture"=0.0, "zoom"=0.0, "field of view"=0.0, "Frame Size"=0, "AOL x centre"=0.0, "AOL y centre"=0.0, "Stage x position"=0.0, "Stage y position"=0.0, "Stage z position"=0.0}, "Z Start"=0.0, "Z Stop"=0.0, "No of Planes"=0, "Laser Power (%) at Z Start"=0.0, "Laser Power (%) at Z Stop"=0.0}, "AOL Z-STACK"={"Hdr Basic Image meta data"={"Wavelength (nm)"=0.0, "# averaged frames"=0.0, "laser power (%)"=0.0, "Pockels"=0.0, "pixel dwell time (us)"=0.0, "pmt 1"=0.0, "pmt 2"=0.0, "back apperture"=0.0, "zoom"=0.0, "field of view"=0.0, "Frame Size"=0, "AOL x centre"=0.0, "AOL y centre"=0.0, "Stage x position"=0.0, "Stage y position"=0.0, "Stage z position"=0.0}, "Z Start"=0.0, "Z Stop"=0.0, "No of Planes"=0, "Laser Power (%) at Z Start"=0.0, "Laser Power (%) at Z Stop"=0.0}, "FUNCTIONAL IMAGING"={"Functional Mode"=enum."Point", "Variable Length"=FALSE, "Variable Resolution"=FALSE, "Pockels Modulation"=FALSE, "Stimuli Trigger"=FALSE, "Cool down enabled"=FALSE, "AOL Mode"=enum."Raster", "Plane Mode"=0, "Miniscan Dwell time per pixel (us)"=0.0, "poi dwell time"=0.0, "Number of trials"=0.0, "Number of cycles"=0.0, "Number of pois"=0.0, "Number of miniscans"=0.0, "Number of pixels in miniscan"=0.0, "Rectangle ROI length"=0.0, "Rectangle ROI height"=0.0, "Frame rate (fps)"=0.0, "Acquisition Length"=0.0, "video length (sec)"=0.0, "Stimuli delay (sec)"=0.0, "Cool down time (sec)"=0.0, "Basic Image meta data"={"Wavelength (nm)"=0.0, "# averaged frames"=0.0, "laser power (%)"=0.0, "Pockels"=0.0, "pixel dwell time (us)"=0.0, "pmt 1"=0.0, "pmt 2"=0.0, "back apperture"=0.0, "zoom"=0.0, "field of view"=0.0, "Frame Size"=0, "AOL x centre"=0.0, "AOL y centre"=0.0, "Stage x position"=0.0, "Stage y position"=0.0, "Stage z position"=0.0}, "Z Start (um)"=0.0, "Z Stop (um)"=0.0}, "VOLUME IMAGING"={"Functional Mode"=enum."Point", "Variable Length"=FALSE, "Variable Resolution"=FALSE, "Pockels Modulation"=FALSE, "Stimuli Trigger"=FALSE, "Cool down enabled"=FALSE, "AOL Mode"=enum."Raster", "Plane Mode"=0, "Miniscan Dwell time per pixel (us)"=0.0, "poi dwell time"=0.0, "Number of trials"=0.0, "Number of cycles"=0.0, "Number of pois"=0.0, "Number of miniscans"=0.0, "Number of pixels in miniscan"=0.0, "Rectangle ROI length"=0.0, "Rectangle ROI height"=0.0, "Frame rate (fps)"=0.0, "Acquisition Length"=0.0, "video length (sec)"=0.0, "Stimuli delay (sec)"=0.0, "Cool down time (sec)"=0.0, "Basic Image meta data"={"Wavelength (nm)"=0.0, "# averaged frames"=0.0, "laser power (%)"=0.0, "Pockels"=0.0, "pixel dwell time (us)"=0.0, "pmt 1"=0.0, "pmt 2"=0.0, "back apperture"=0.0, "zoom"=0.0, "field of view"=0.0, "Frame Size"=0, "AOL x centre"=0.0, "AOL y centre"=0.0, "Stage x position"=0.0, "Stage y position"=0.0, "Stage z position"=0.0}, "Z Start (um)"=0.0, "Z Stop (um)"=0.0}, "MOVEMENT CORRECTION"={"Movement Correction"=FALSE, "Axial Reference"=FALSE, "Reference Source"=enum."Green channel", "Full Frame Size"=0.0, "Reference Field of View"=0.0, "Reference Zoom"=0.0, "Reference dwell time (us)"=0.0, "Reference X Pixels"=0.0, "Reference Y Pixels"=0.0, "Number of Z lines"=0.0, "Size of Z pixels"=0.0, "Axial Pixels"=0.0, "Ignore Z lines"=0.0, "Reference Scan Cycles"=0.0, "Reference Threshold XY"=0.0, "Reference Threshold Z"=0.0, "Reference Average XY"=0.0, "Reference Average Z"=0.0, "Proportional Scale"=0.0, "Integral Scale"=0.0, "Proportional Scale Z"=0.0, "Integral Scale Z"=0.0, "Diff Threshold"=0.0, "Diff Threshold Z"=0.0, "Sliding Average"=FALSE, "Reference count reset enabled"=FALSE, "Scan Interval (ms)"=0.0, "Ref Plot Refresh Rate (ms)"=0.0}, "CALIBRATION"={"Pockels Calibration File"=path "", "Calibration_ini file"=path "", "Setup_ini file"=path ""}, "STATISTICS"={"Z-stack duration (sec)"=0.0, "Number of acquired data-points"=0.0, "Acquisition time (ms)"=0.0, "Number of acquired frames"=0.0, "Intertrial times"=[]}, "BIOLOGY INFORMATION"={"Animal Code or Name"="", "Animal DoB"="", "Animal Age"="", "Animal Sex"="", "Animal Weight"="", "Date of Injection"="", "Date of Implant"="", "Site of Injection"="", "Animal Ear Notch"="", "AAV constructs"="", "Genetic background"="", "Optical reporter"="", "Region of brain imaged"="", "Other \ncomments"=""}, "Calibration Data"={"Objective Name"="", "Calibration Wavelength"=0.0, "Sum X"=0.0, "Sum Y"=0.0, "Diff X"=0.0, "Diff Y"=0.0, "Distortion Correction"=0.0, " Z norm to um Scaling"=0.0, " X norm to um Scaling"=0.0}} ("All header parameters in"), "BIOLOGY INFORMATION"=w224) -> (w223:T6)
    }
  }
  "All header parameters in" <- w1
  n100 = case shown="True" "Update header\ninterface cluster ?" {
    tunnel: w1 -> [_ w231]
    tunnel: "error in (no error)" -> [w227 w230]
    tunnel: [w227 w229] -> w5
    tunnel: "Header file sections" -> [_ w228]
    frame False {
    }
    frame True {
      n101 = call "Experiment header-Interface module.vi"("Header file sections"=w228, "error in (no error)"=w230, "All header parameters in"=w231, "Function"=Header_file_interface_module_functions_enum."Update values in memory") -> ("error out"=w229:errorcluster)  [unwired: 6 in, 1 out]
    }
  }
  "error out" <- w5
